vi "EnFlo_Hub.vi"() -> ()   [LabVIEW 2015]
uses:
  Anemometry Sub Vis/Controls/Launch_controls/Open_Calib.ctl
  Anemometry Sub Vis/Controls/Launch_controls/Open_Meas.ctl
  Anemometry Sub Vis/Controls/Launch_controls/Open_Enter_Temp.ctl
  Anemometry Sub Vis/Controls/Launch_controls/Multi_Run_Prog.ctl
  Anemometry Sub Vis/Controls/Launch_controls/EnFlo_arm.ctl
  Anemometry Sub Vis/Controls/Launch_controls/Fast_FID_Valve.ctl
  Anemometry Sub Vis/Controls/Launch_controls/Disp_Setup.ctl
  Anemometry Sub Vis/Controls/Launch_controls/EnFlo_Tun_Setup.ctl
  Anemometry Sub Vis/Controls/Launch_controls/User_Metadata.ctl
  Anemometry Sub Vis/Controls/Launch_controls/Trav_3D_move.ctl
  Anemometry Sub Vis/Controls/Launch_controls/Trav_Space.ctl
  Anemometry Sub Vis/Controls/Launch_controls/Tunnel_speed.ctl
  Anemometry Sub Vis/Controls/Launch_controls/Client_source_control.ctl
  Anemometry Sub Vis/Controls/Launch_controls/Hydrosonic_Manual.ctl
  Anemometry Sub Vis/Controls/Launch_controls/Preference_Panel.ctl
  Anemometry Sub Vis/Controls/Launch_controls/Hot_wire_Calculator.ctl
  Anemometry Sub Vis/Controls/Launch_controls/RW_X_Parker_Config.ctl
  Anemometry Sub Vis/Controls/Launch_controls/LDA_Alignment.ctl
  Anemometry Sub Vis/Controls/Launch_controls/Named_Serial_Comms.ctl
  Anemometry Sub Vis/Controls/Launch_controls/BSA_data_rates.ctl
  Anemometry Sub Vis/Controls/Launch_controls/Serial_Setup.ctl
  Anemometry Sub Vis/Controls/Launch_controls/Post_Process_icon.ctl
  Anemometry Sub Vis/Controls/Launch_controls/Edit_Ascii_file.ctl
  Anemometry Sub Vis/Controls/Launch_controls/Edit_Raw_DF.ctl
  Anemometry Sub Vis/Controls/Launch_controls/Results_file_plotter.ctl
  Anemometry Sub Vis/Controls/Launch_controls/Serial_Port_Names.ctl
  Anemometry Sub Vis/Controls/Launch_controls/Paul.ctl
  Anemometry Sub Vis/Controls/Launch_controls/Tom.ctl
  Anemometry Sub Vis/Controls/Launch_controls/Scani_Valve.ctl
  Anemometry Sub Vis/Controls/Launch_controls/Edit_sever_Channel.ctl
  Anemometry Sub Vis/Controls/Launch_controls/Day_file_plotter.ctl
  Anemometry Sub Vis/Controls/Launch_controls/Plot_Sever_Data.ctl
  Anemometry Sub Vis/Controls/Launch_controls/Adam_Table.ctl
  Anemometry Sub Vis/Controls/Launch_controls/Active_Channel_Control.ctl
  Anemometry Sub Vis/Controls/Launch_controls/Laser on,off.ctl
  Anemometry Sub Vis/Controls/Launch_controls/Laser set power.ctl
  Anemometry Sub Vis/Controls/Preference_Mode.ctl
  Anemometry Sub Vis/Controls/Post_Process.ctl
  Anemometry Sub Vis/Controls/Setup.ctl
  Anemometry Sub Vis/Gen Trav/Trav_mode.ctl
  Anemometry Sub Vis/Controls/User_Specific_mode.ctl
  Anemometry Sub Vis/File/Setup_Filetype.ctl
  Anemometry Sub Vis/Calibration/Calib_mode.ctl
  Anemometry Sub Vis/Controls/Server_Comms.ctl
  ADAM Client/Sub VIs/ADAM Controls/Update_scan_value.ctl
  Anemometry Sub Vis/Controls/App_Global.ctl
  Anemometry Sub Vis/Globals/Meas_global.vi
  Anemometry Sub Vis/Globals/Dynamic_call_global.ph.vi
  Anemometry Sub Vis/Globals/Trav_pos_global.vi
  Anemometry Sub Vis/Globals/Constants_global.vi
  Anemometry Sub Vis/Globals/Preference_global.vi
  Anemometry Sub Vis/Acquisition/PWA/PWAtasksGLOBAL.vi
  <vilib>/Platform/browser.llb/Open URL in Default Browser (string).vi
  Anemometry Sub Vis/Utilities/Email_transfer_global.vi
  Camera Server/Globals/CamServer global.vi
panel:
  out "CamServer machine name or IP":string="EnFlo-CamServer"
  out "List of ADAM channels to view":string[](array[string])
  out "List of ADAM control channels":string[](array[string])
  out "Analogue Dev Name":string="Dev2"
  out "Numeric":i32
  out "Rig Name":string="EnFlo Tunnel"
  out "All Users":path=path "/System Folder/Preferences/LabVIEW (EnFlo specific)/Meas Setups"
  out "Dummy Measurement":bool
  in  "stop":bool
  in  "Tab Control":T1(tab)
  in  "Tunnel Speed Control":T2
  in  "Traverse Space":T3
  in  "Trav 3D Move":T4 caption="3D Traverse Move"
  in  "User Metadata":T5
  in  "Multi Run Prog":T6
  in  "Enter Temp_Press":T7
  in  "Measurement Prog":T8 caption="Measurement"
  in  "Calibration Prog":T9 caption="Calibration"
  in  "Source Live":bool
  in  "Laser set power":T10
  in  "Laser on/off":T11
  in  "Scani Valve":T12
  in  "LDA Alignment":T13
  in  "Hydrosonic Control":T14
  in  "Fast FID Valve":T15
  in  "Source Control":T16
  in  "Gas Release Setup":T17
  in  "EnFlo Tunnel Setup":T18
  in  "Heater Setup":bool caption="Inlet heater File"
  in  "EnFlo Arm":T19
  in  "EnFlo Tun Display":bool
  in  "Beam Check Positions":bool
  in  "Rig_Control":cluster{"Ch Name":string, "Boolean":bool}[](array[cluster])
  in  "ADAM Channels Control":T20 caption="Change Active Channels"
  in  "ADAM Scan Table":T21 caption="Run ADAM Scan Table"
  in  "Edit Server Channel":T22
  in  "Plot Server Channels":T23 caption="Plot Server Data"
  in  "Day Files Plotter":T24 caption="Plot Data From File"
  out "Current Values":cluster{"Ch Name":string, "Numeric":dbl}[](array[cluster])
  in  "Post_Pro_Results_Hierarchy":bool
  in  "Results File Plotter":T25
  in  "Edit Raw Data Files":T26
  in  "Edit ASCII File":T27
  in  "Post Process Raw Data":T28
  in  "Plot_FFID_Calibs.vi":bool
  in  "Top Level Traverse":bool
  in  "Show Manual Sync":bool
  in  "Sync to server now":bool
  in  "Port Names":T29
  in  "Serial Setup":T30
  in  "LDA Data Rate":T31
  in  "Named Serial Comms":T32
  in  "RW Trav Setup":T33
  in  "Hot Wire Calc":T34
  in  "Preference Panel":T35
  in  "Tom Lawton tlawton@cppwind.com":T36 caption="For -other- support"
  in  "Paul Hayden p.hayden@surrey.ac.uk":T37 caption="For software support"
  in  "Online Manual":bool
  out "VI Name":string
  out "Iterations":i32
  # "Or give us a call on Tel: 01483 689545"
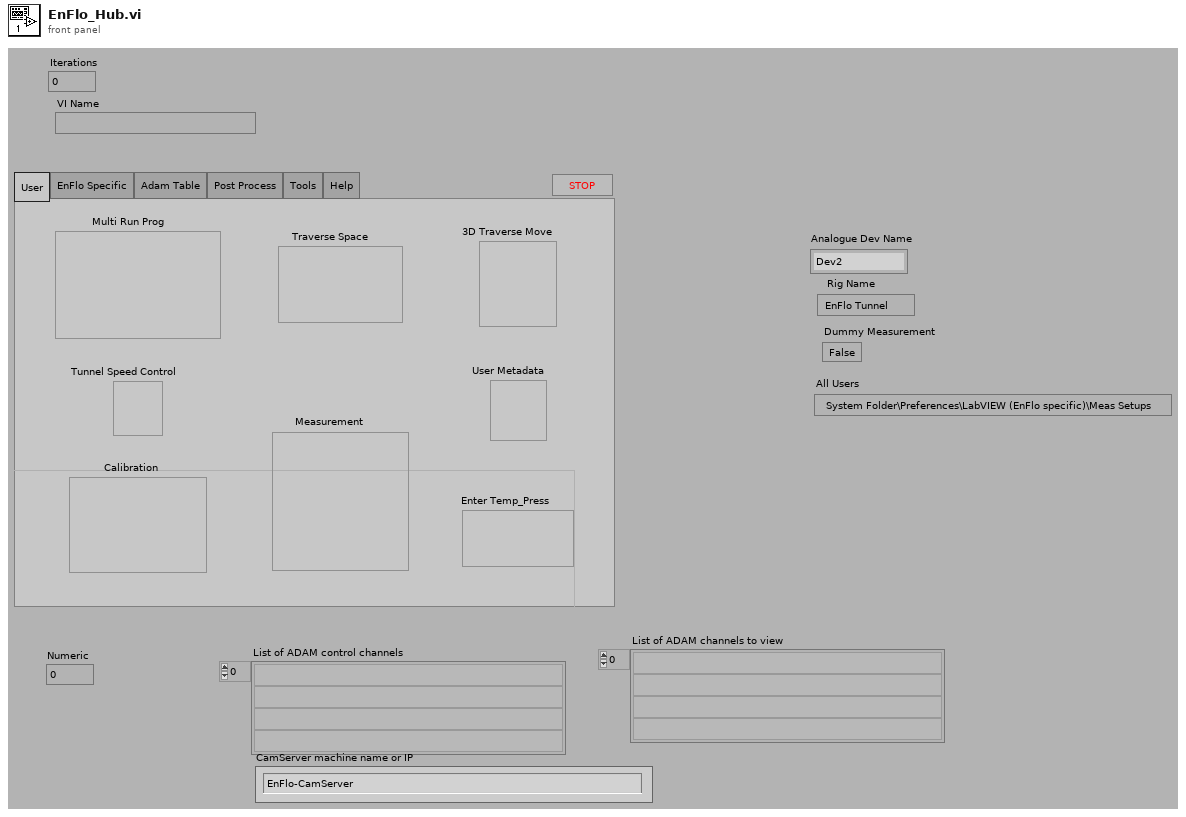
[diagram p1: front panel]
types:
  T1 = enum32{"User", "EnFlo Specific", "Adam Table", "Post Process", "Tools", "Help"}
  T2 = typedef "Tunnel_speed.ctl" = bool
  T3 = typedef "Trav_Space.ctl" = bool
  T4 = typedef "Trav_3D_move.ctl" = bool
  T5 = typedef "User_Metadata.ctl" = bool
  T6 = typedef "Multi_Run_Prog.ctl" = bool
  T7 = typedef "Open_Enter_Temp.ctl" = bool
  T8 = typedef "Open_Meas.ctl" = bool
  T9 = typedef "Open_Calib.ctl" = bool
  T10 = typedef "Laser set power.ctl" = bool
  T11 = typedef "Laser on,off.ctl" = bool
  T12 = typedef "Scani_Valve.ctl" = bool
  T13 = typedef "LDA_Alignment.ctl" = bool
  T14 = typedef "Hydrosonic_Manual.ctl" = bool
  T15 = typedef "Fast_FID_Valve.ctl" = bool
  T16 = typedef "Client_source_control.ctl" = bool
  T17 = typedef "Disp_Setup.ctl" = bool
  T18 = typedef "EnFlo_Tun_Setup.ctl" = bool
  T19 = typedef "EnFlo_arm.ctl" = bool
  T20 = typedef "Active_Channel_Control.ctl" = bool
  T21 = typedef "Adam_Table.ctl" = bool
  T22 = typedef "Edit_sever_Channel.ctl" = bool
  T23 = typedef "Plot_Sever_Data.ctl" = bool
  T24 = typedef "Day_file_plotter.ctl" = bool
  T25 = typedef "Results_file_plotter.ctl" = bool
  T26 = typedef "Edit_Raw_DF.ctl" = bool
  T27 = typedef "Edit_Ascii_file.ctl" = bool
  T28 = typedef "Post_Process_icon.ctl" = bool
  T29 = typedef "Serial_Port_Names.ctl" = bool
  T30 = typedef "Serial_Setup.ctl" = bool
  T31 = typedef "BSA_data_rates.ctl" = bool
  T32 = typedef "Named_Serial_Comms.ctl" = bool
  T33 = typedef "RW_X_Parker_Config.ctl" = bool
  T34 = typedef "Hot_wire_Calculator.ctl" = bool
  T35 = typedef "Preference_Panel.ctl" = bool
  T36 = typedef "Tom.ctl" = bool
  T37 = typedef "Paul.ctl" = bool
  T38 = typedef "Post_Process.ctl" = enum16{"Take New Data", "Post Process Raw Data File"}
  T39 = typedef "Preference_Mode.ctl" = enum16{"Load Preferences from file", "Save Preferences to file", "Load, Edit then Save"}
  T40 = enum32{"User", "EnFlo Lab Specific", "Adam Table", "Post Process", "Tools", "Help"}
  T41 = typedef "Server_Comms.ctl" = enum16{"Server Link Healthy", "Do Not Link To Server"}
  T42 = typedef "Update_scan_value.ctl" = cluster{"Channel Name":string, "New Value":dbl}
  T43 = typedef "Setup.ctl" = enum16{"Run Program", "Show Setup", "Save Current Setup", "Setup Front Panel"}
  T44 = enum16{"Get Channel Names", "Get Current Value", "Update Channel Value", "Update Channel Description"}
  T45 = enum32{"Invalid", "Standard", "Closed", "Hidden", "Minimized", "Maximized"}
  T46 = enum32{"Bad", "Idle", "Run top level", "Running"}
  T47 = enum16{"Load From Excel File", "Save to Excel File"}
  T48 = typedef "User_Specific_mode.ctl" = enum16{"Check VI only", "Run VI"}
  T49 = typedef "Trav_mode.ctl" = enum16{"Move traverse", "Read traverse position", "Teach Position"}
  T50 = typedef "Setup_Filetype.ctl" = enum16{"Measurement Setups", "Calibration Setups", "General", "Results File Plotter Setups", "Speed Calib Tweaks"}
  T51 = enum16{"Load Command File", "Save Command File", "Check Multi Run Prog", "Check Multi Run Prog With Live Moves", "Run Multi Run Prog"}
  T52 = typedef "Calib_mode.ctl" = enum16{"Show Setup", "Take a New Calibration Point", "Refit Curve", "Setup Front Panel"}
  T53 = typedef "App_Global.ctl" = enum16{"Read Global", "Write to Global", "Initialise Array"}
  T54 = typedef "Tunnel_Coordinates.ctl" = enum16{"Work in Tunnel Coordinates", "Work in Model Coordinates"}
  T55 = typedef "App_Ref_Cluster.ctl" = cluster{"Server IP & Port No":string, "Application reference":refnum<vi>}
  T56 = typedef "Ch_description_ADAM.ctl" = cluster{"Ch Name":string, "Type":T57, "Function":T58, "Ch State":T59, "Calibration type":T60, "A":dbl, "B":dbl, "C":dbl, "D":dbl, "Comments":string, "Address":T61, "String":string, "Duty":u16}
  T57 = typedef "Module_type_ADAM.ctl" = string
  T58 = typedef "Function_ADAM.ctl" = enum16{"Analogue Input", "Digital Input", "Event counter", "Event rate", "Analogue Output", "Digital Output", "Relay Output"}
  T59 = typedef "Channel_State.ctl" = enum16{"On", "Off", "Always On", "Always Off"}
  T60 = typedef "Calib_type_ADAM.ctl" = enum16{"Raw", "Bx + A", "Cx^2 + Bx + A", "Dx^3 + Cx^2 + Bx + A", "In Band", "Hi-Tec Q", "Hi-Tec M_dot", "Text"}
  T61 = typedef "Address.ctl" = cluster{"Main":i32, "Ch.":i32, "Sub":i32, "Port Name":string}
  T62 = typedef "Monitor values.ctl" = cluster{"Power (mW)":sgl, "LDD current (A)":sgl, "TEC drive (V)":sgl, "TEC temp. (degC)":sgl, "SHG heater (degC)":sgl, "BRF heater (degC)":sgl}
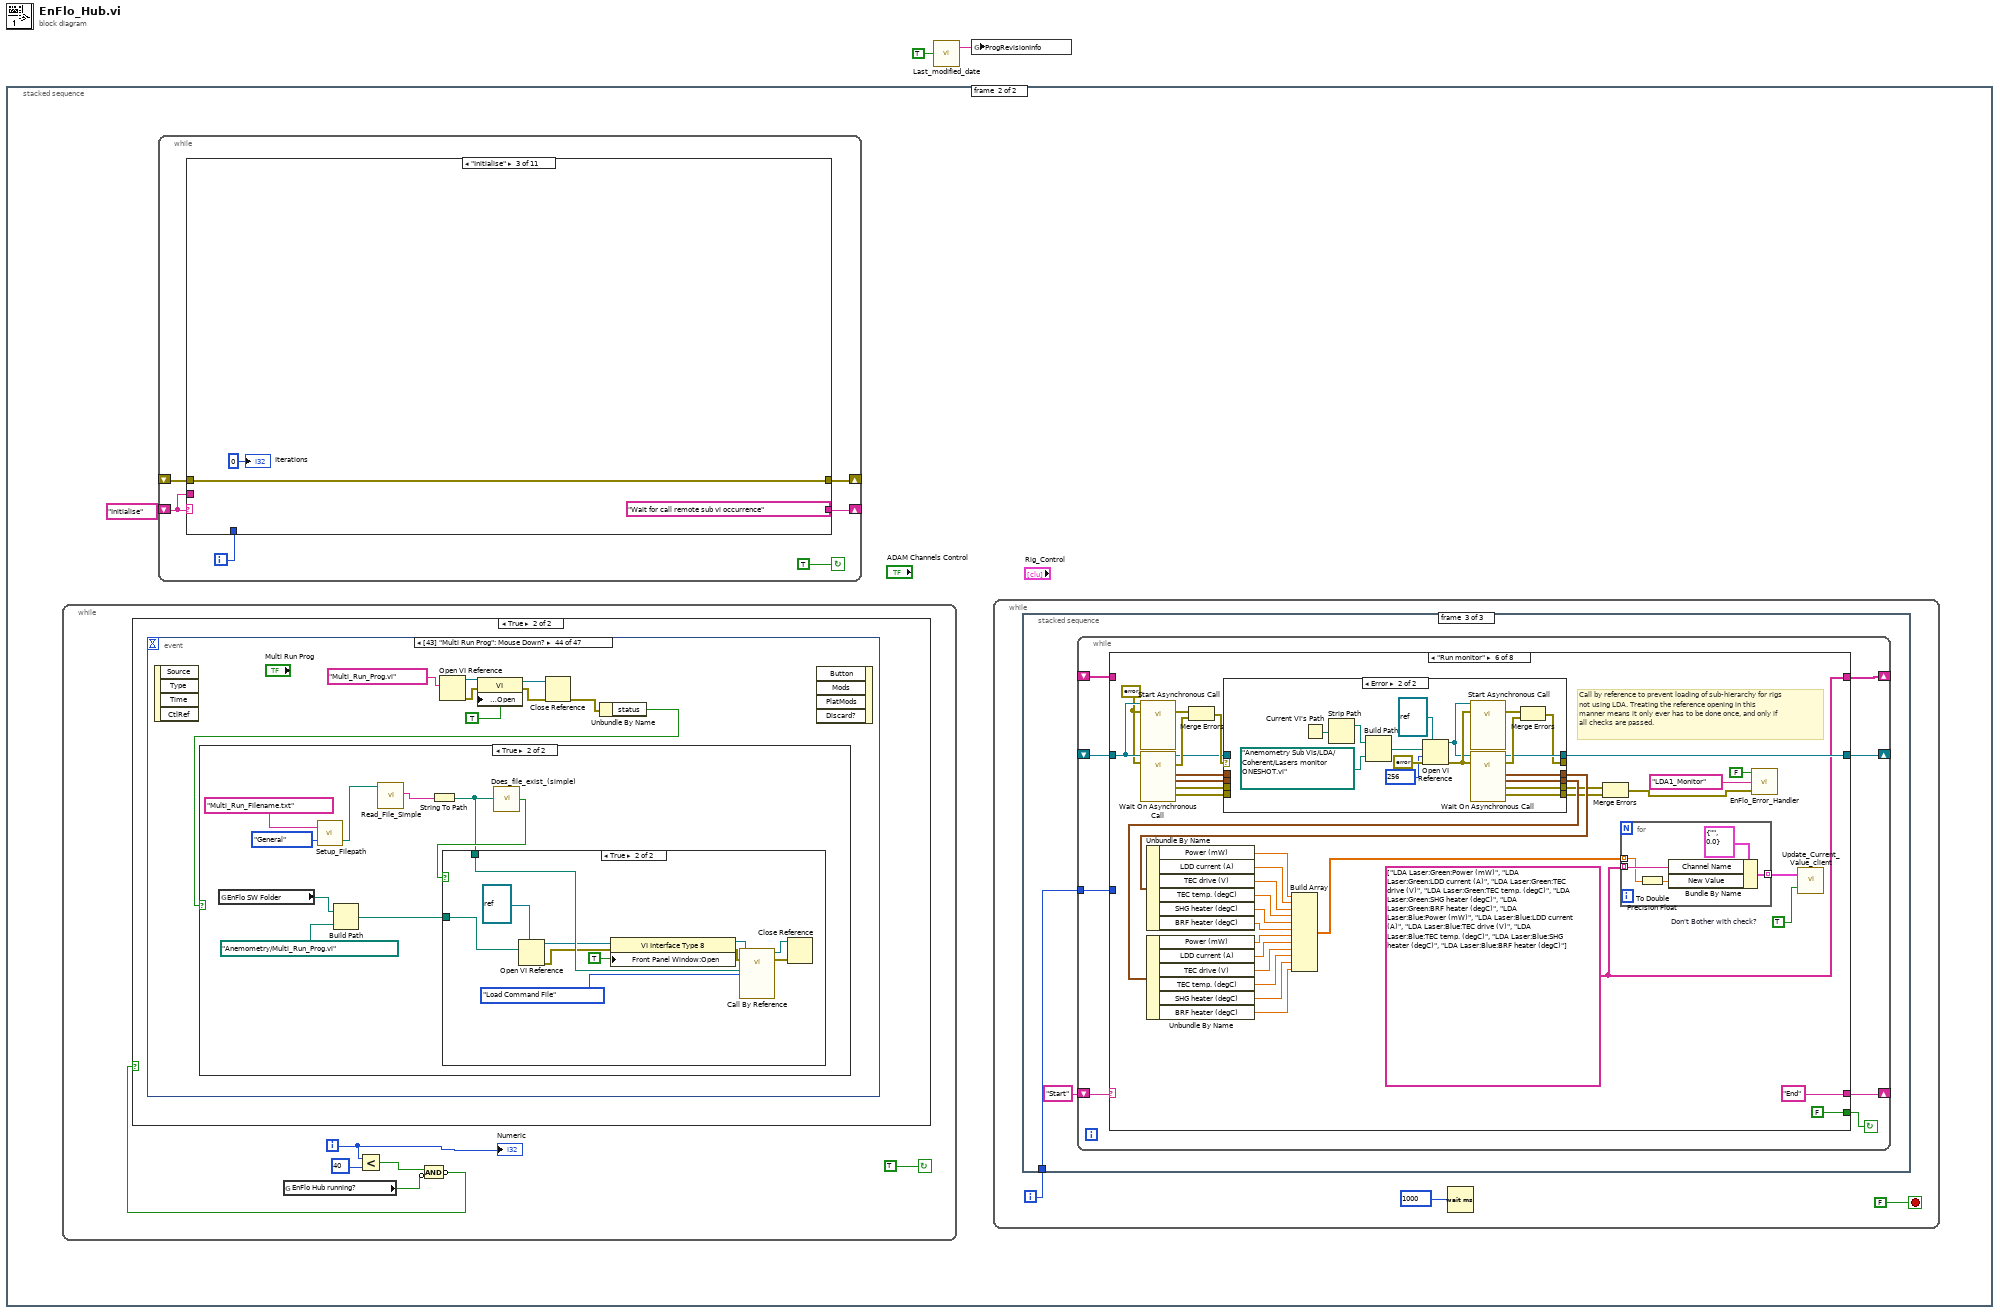
[diagram p0: block diagram]
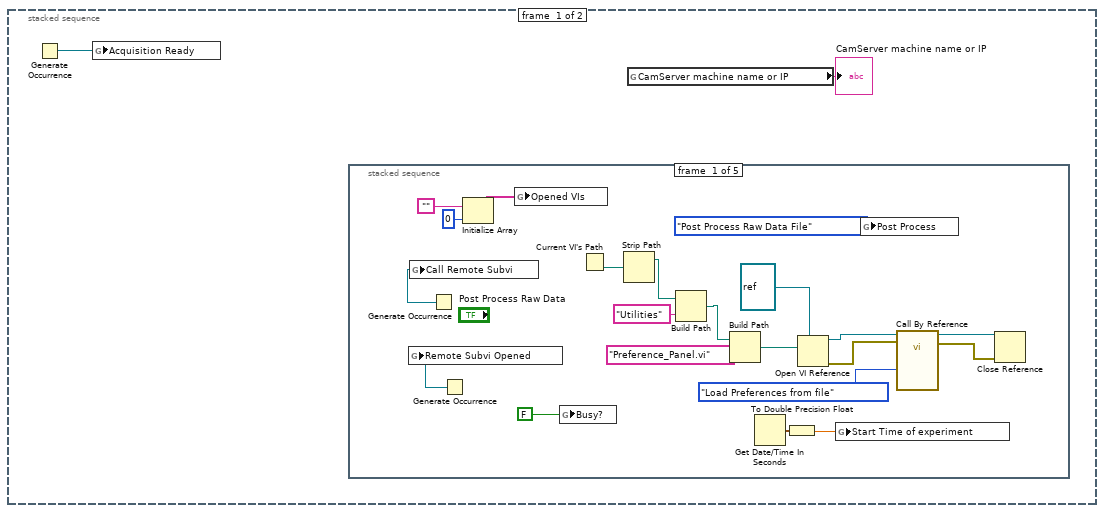
[diagram p2: hidden frame]
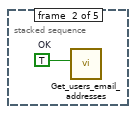
[diagram p3: hidden frame]
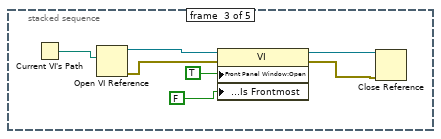
[diagram p4: hidden frame]
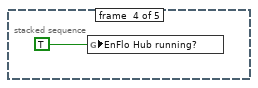
[diagram p5: hidden frame]
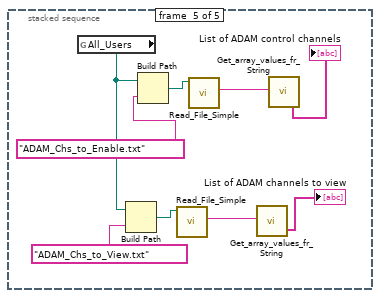
[diagram p6: hidden frame]
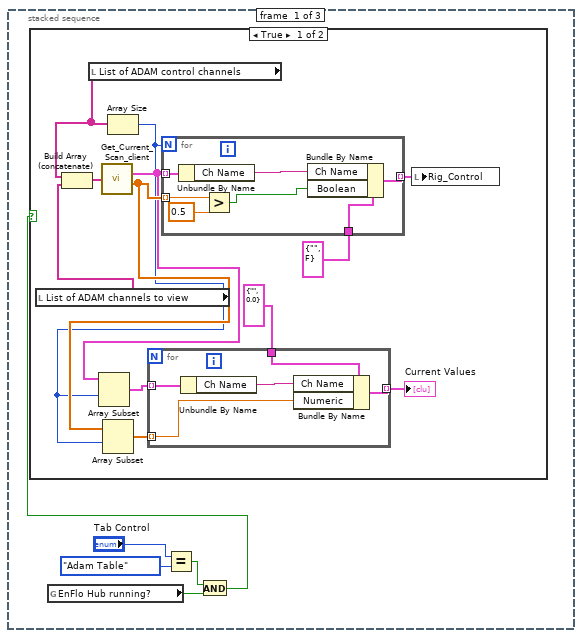
[diagram p7: hidden frame]
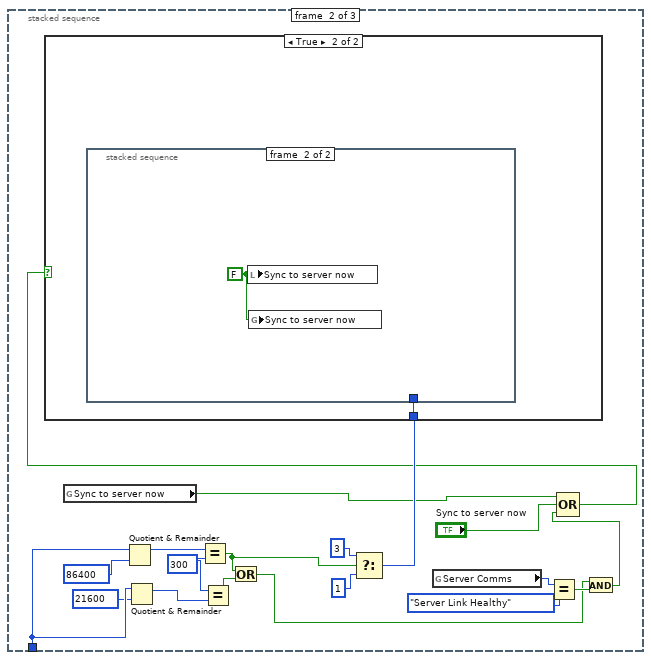
[diagram p9: hidden frame]
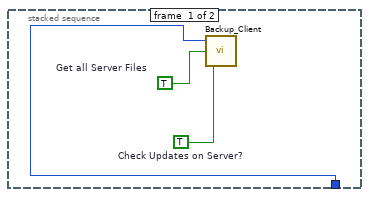
[diagram p11: hidden frame]
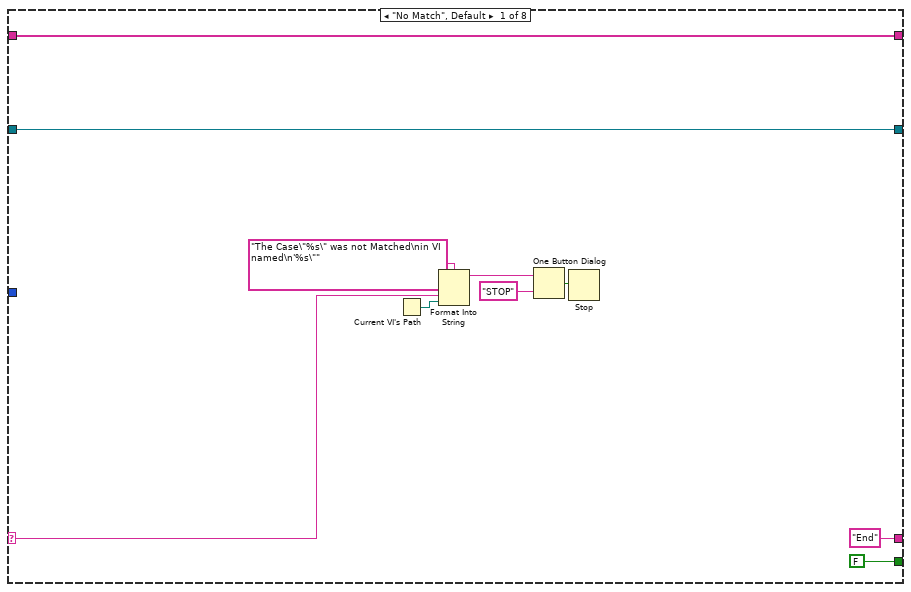
[diagram p12: hidden frame]
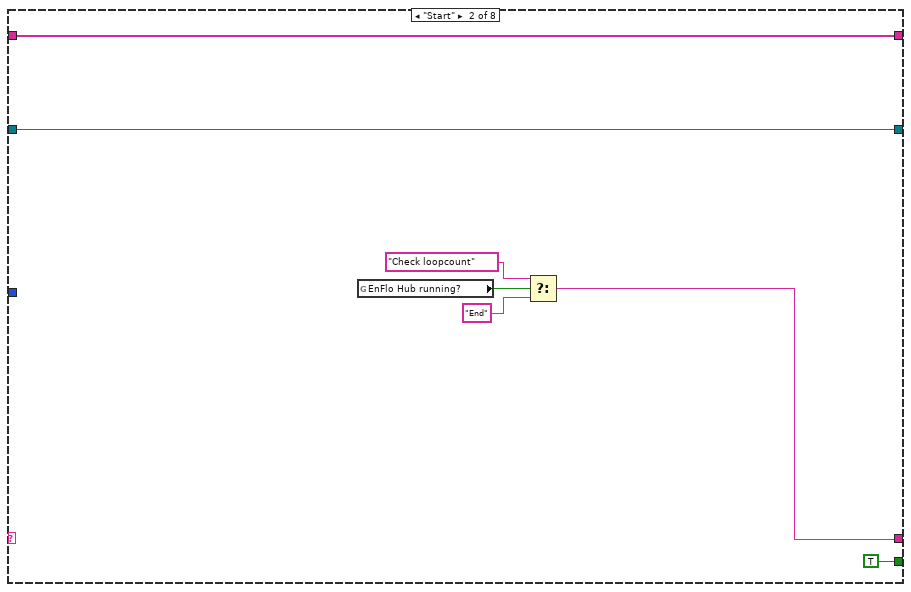
[diagram p13: hidden frame]
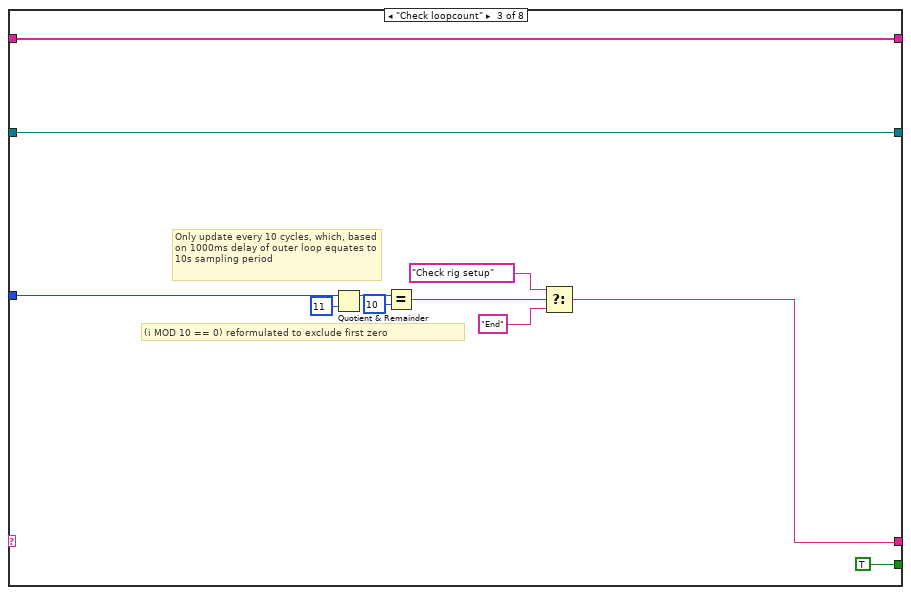
[diagram p14: hidden frame]
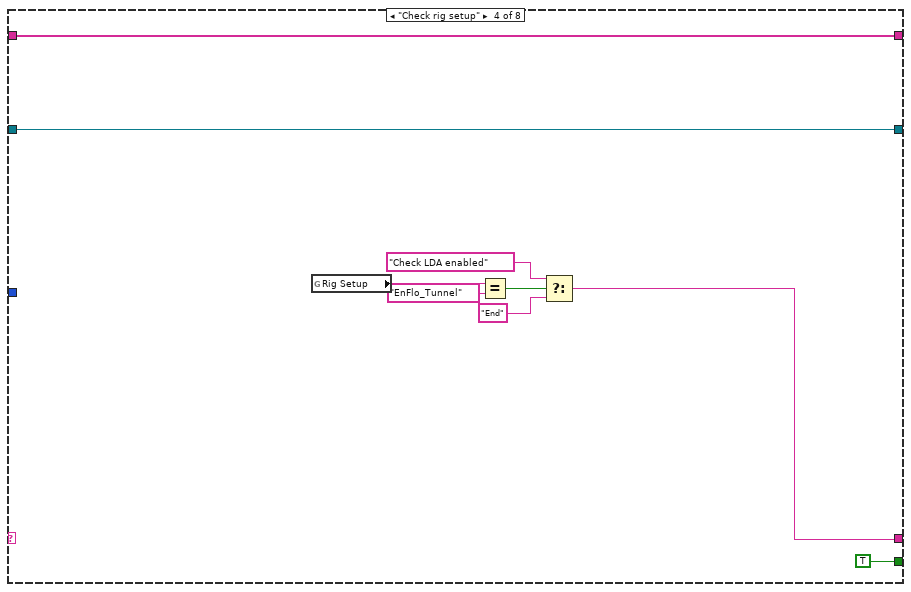
[diagram p15: hidden frame]
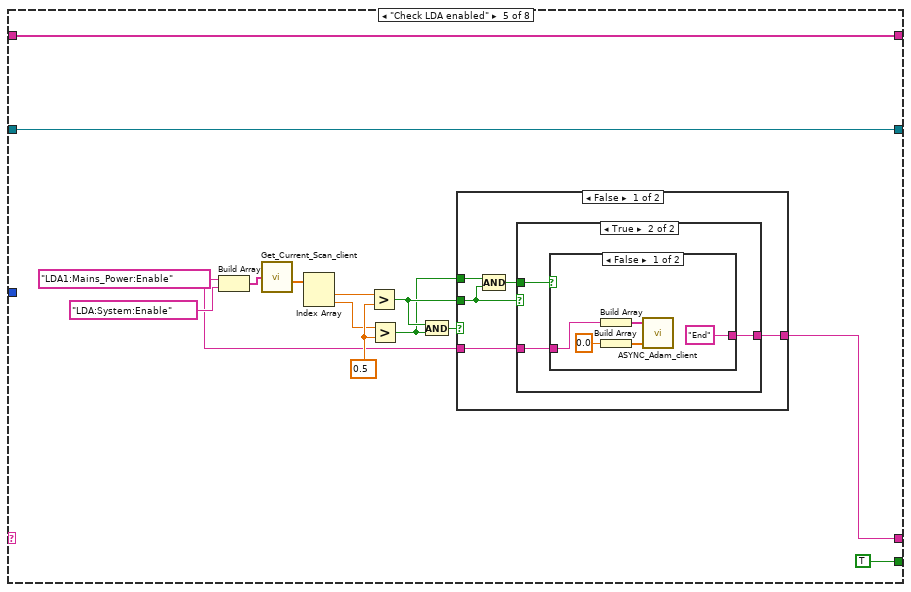
[diagram p16: hidden frame]
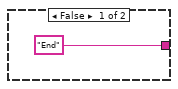
[diagram p17: hidden frame]
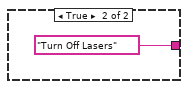
[diagram p18: hidden frame]
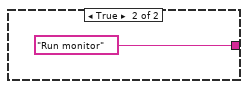
[diagram p19: hidden frame]
diagram:
  n1 = stacked-sequence {
    frame #0 {
      n2 = Generate Occurrence() -> (w4:refnum<k4>)
      n3 = global write "Meas_global.vi" "Acquisition Ready"(w4) -> ()
      n4 = stacked-sequence {
        frame #0 {
          n5 = Generate Occurrence() -> (w25:refnum<k4>)
          n6 = global write "Dynamic_call_global.ph.vi" "Call Remote Subvi"(w25) -> ()
          n7 = Generate Occurrence() -> (w24:refnum<k4>)
          n8 = global write "Dynamic_call_global.ph.vi" "Remote Subvi Opened"(w24) -> ()
          n9 = Initialize Array("", 0) -> (w22:string[])
          n10 = global write "Dynamic_call_global.ph.vi" "Opened VIs"(w22) -> ()
          n11 = global write "Email_transfer_global.vi" "Busy?"(FALSE ("Busy?")) -> ()
          n12 = Current VI's Path() -> (path=w14:path)
          n13 = Strip Path(path=w14) -> (stripped path=w12:path)  [unwired: 1 out]
          n14 = Build Path(base path=w12, name or relative path="Utilities") -> (appended path=w10:path)
          n15 = Build Path(base path=w10, name or relative path="Preference_Panel.vi") -> (appended path=w9:path)
          n16 = Get Date/Time In Seconds() -> (seconds since 1Jan1904=w20:timestamp)
          n17 = To Double Precision Float(number=w20) -> (double precision float=w19:dbl)
          n18 = Open VI Reference(type specifier VI Refnum (for type only)=refnum<vi> refnum, vi path=w9) -> (vi reference=w15:refnum<vi>, error out=w16:errorcluster)  [unwired: 1 in, 3 out]
          n19 = global write "Meas_global.vi" "Start Time of experiment"(w19) -> ()
          n20 = global write "Meas_global.vi" "Post Process"(Post_Process."Post Process Raw Data File" ("Post Process")) -> ()
          n21 = call-by-ref "?"(reference=w15, error in=w16, "Mode"=Preference_Mode."Load Preferences from file") -> (reference out=w17:refnum<vi>, error out=w18:errorcluster)
          n22 = Close Reference(reference=w17, error in (no error)=w18) -> ()  [unwired: 1 out]
        }
        frame #1 {
          w26 = TRUE  # OK
          n23 = call "Get_users_email_addresses.vi"("OK"=w26) -> ()  [unwired: 5 out]
        }
        frame #2 {
          n24 = Current VI's Path() -> (path=w33:path)
          n25 = Open VI Reference(vi path=w33) -> (vi reference=w32:refnum<vi>, error out=w31:errorcluster)  [unwired: 1 in, 4 out]
          n26 = property class="VI"(reference=w32, error in=w31, "Front Panel Window:Open"=TRUE, "Front Panel Window:Is Frontmost"=FALSE) -> (reference out=w30:refnum<vi>, error out=w29:errorcluster)
          n27 = Close Reference(reference=w30, error in (no error)=w29) -> ()  [unwired: 1 out]
        }
        frame #3 {
          n28 = global write "Dynamic_call_global.ph.vi" "EnFlo Hub running?"(TRUE ("EnFlo Hub running?")) -> ()
        }
        frame #4 {
          n29 = global read "Constants_global.vi" "All_Users"() -> (w38:path)
          n30 = Build Path(base path=w38, name or relative path="ADAM_Chs_to_View.txt") -> (appended path=w40:path)
          n31 = Build Path(base path=w38, name or relative path="ADAM_Chs_to_Enable.txt") -> (appended path=w42:path)
          n32 = call "Read_File_Simple.vi"("Filename"=w40) -> ("string"=w39:string)  [unwired: 2 in, 7 out]
          n33 = call "Read_File_Simple.vi"("Filename"=w42) -> ("string"=w43:string)  [unwired: 2 in, 7 out]
          n34 = call "Get_array_values_fr_String.vi"("String Value"=w39) -> ("String array"=→"List of ADAM channels to view":string[])  [unwired: 1 out]
          n35 = call "Get_array_values_fr_String.vi"("String Value"=w43) -> ("String array"=→"List of ADAM control channels":string[])  [unwired: 1 out]
        }
      }
      n36 = global read "CamServer global.vi" "CamServer machine name or IP"() -> (→"CamServer machine name or IP":string)
    }
    frame #1 {
      n37 = while {
        i -> [w272]
        stop <- TRUE continue-if-true
        n38 = global read "Dynamic_call_global.ph.vi" "EnFlo Hub running?"() -> (w270:bool)
        n39 = Less?(x=w272, y=40) -> (x < y?=w269:bool)
        n40 = Compound Arithmetic op=AND(w269, invert w270) -> (invert w268:bool)
        n41 = case shown="True" w268 {
          frame False {
            n42 = Wait (ms)(milliseconds to wait=u32 200) -> ()  [unwired: 1 out]
          }
          frame True {
            n43 = event shown="[43] \"Multi Run Prog\": Mouse Down?" {
              selector: _ -> [_ _ _ _ _ _ _ _ _ _ _ _ _ _ _ _ _ _ _ _ _ _ _ _ _ _ _ _ _ _ _ _ _ _ _ _ _ _ _ _ _ _ _ _ _ _ _]
              dyn-events: _ -> [_ _ _ _ _ _ _ _ _ _ _ _ _ _ _ _ _ _ _ _ _ _ _ _ _ _ _ _ _ _ _ _ _ _ _ _ _ _ _ _ _ _ _ _ _ _ _]
              timeout: _ -> [_ _ _ _ _ _ _ _ _ _ _ _ _ _ _ _ _ _ _ _ _ _ _ _ _ _ _ _ _ _ _ _ _ _ _ _ _ _ _ _ _ _ _ _ _ _ _]
              event Mouse Down? {
                w283 = "Measurement.vi" ("name or relative path")
                n44 = event-data() -> ()  [unwired: 2 out]
                n45 = global read "Constants_global.vi" "EnFlo SW Folder"() -> (w286:path)
                n46 = Open VI Reference(vi path=w283) -> (vi reference=w282:refnum<vi>, error out=w281:errorcluster)  [unwired: 1 in, 4 out]
                n47 = Build Path(base path=w286, name or relative path="Anemometry") -> (appended path=w289:path)
                n48 = property class="VI"(reference=w282, error in=w281, "Front Panel Window:Open"=TRUE) -> (reference out=w279:refnum<vi>, error out=w280:errorcluster)
                n49 = Build Path(base path=w289, name or relative path=w283) -> (appended path=w287:path)
                n50 = global read "Preference_global.vi" "Rig Setup"() -> (w277:string)
                n51 = Close Reference(reference=w279, error in (no error)=w280) -> (error out=w278:errorcluster)
                n52 = Unbundle By Name(w278) -> ("status"=w288:bool)
                n53 = Equal?(x="Post_Processing_Machine" ("Rig Setup"), y=w277) -> (x = y?=w275:bool)
                n54 = case shown="True" w288 {
                  tunnel: w287 -> [_ w292]
                  tunnel: w278 -> [_ _]
                  tunnel: w275 -> [_ w291]
                  frame False {
                  }
                  frame True {
                    n55 = stacked-sequence {
                      tunnel: w292 -> [w302 _]
                      tunnel: w291 -> [w293 _]
                      frame #0 {
                        n56 = Open VI Reference(type specifier VI Refnum (for type only)=refnum<vi> refnum, vi path=w302) -> (vi reference=w300:refnum<vi>, error out=w299:errorcluster)  [unwired: 1 in, 3 out]
                        n57 = property class="VI Interface Type 1"(reference=w300, error in=w299, "Front Panel Window:Open"=TRUE) -> (reference out=w295:refnum<vi>, error out=w294:errorcluster)
                        n58 = case shown="False" w293 {
                          tunnel: [w308 w310] -> w298
                          tunnel: [w307 w309] -> w297
                          tunnel: w295 -> [w306 w310]
                          tunnel: w294 -> [w305 w309]
                          frame False {
                            n59 = call-by-ref "?"(reference=w306, error in=w305, "setup"=Setup."Setup Front Panel", "Post Process"=Post_Process."Take New Data") -> (reference out=w308:refnum<vi>, error out=w307:errorcluster)  [unwired: 16 in, 2 out]
                          }
                          frame True {
                          }
                        }
                        n60 = Close Reference(reference=w298, error in (no error)=w297) -> ()  [unwired: 1 out]
                      }
                      frame #1 {
                        n61 = global write "Meas_global.vi" "Post Process"(Post_Process."Post Process Raw Data File" ("Post Process")) -> ()
                      }
                    }
                  }
                }
                n62 = event-data("Discard?"=TRUE) -> ()  [unwired: 1 in, 2 out]
              }
              event Mouse Down? {
                n63 = event-data() -> ()  [unwired: 2 out]
                n64 = call-poly <vilib>:"Open URL in Default Browser.vi"("URL"="Mailto:tlawton@cppwind.com") -> ()  [unwired: 1 in, 6 out]
                n65 = event-data() -> ()  [unwired: 1 in, 5 out]
              }
              event Mouse Down? {
                n66 = event-data() -> ()  [unwired: 5 out]
                n67 = call-poly <vilib>:"Open URL in Default Browser.vi"("URL"="Mailto:p.hayden@surrey.ac.uk") -> ()  [unwired: 1 in, 6 out]
                n68 = event-data() -> ()  [unwired: 1 in, 2 out]
              }
              event "Online Manual": Mouse Down? {
                n69 = event-data() -> ()  [unwired: 2 out]
                n70 = call-poly <vilib>:"Open URL in Default Browser.vi"("URL"="http://131.227.181.18/~xphayden/enflosw/beta/Manual/online/index.html") -> ()  [unwired: 1 in, 6 out]
                n71 = event-data() -> ()  [unwired: 1 in, 2 out]
              }
              event Mouse Down? {
                n72 = event-data() -> ()  [unwired: 9 out]
                n73 = global read "Constants_global.vi" "EnFlo SW Folder"() -> (w315:path)
                n74 = Build Path(base path=w315, name or relative path=path "ADAM Client/ADAM client VIs/ScaniValve_client.vi") -> (appended path=w318:path)
                n75 = call "Open_Close_Front_Panel.ph.vi"("Front Panel Window:Open"=TRUE, "VI path"=w318) -> ()  [unwired: 2 out]
                n76 = event-data() -> ()  [unwired: 1 in, 5 out]
              }
              event Mouse Down? {
                n77 = event-data() -> ()  [unwired: 9 out]
                n78 = global read "Constants_global.vi" "EnFlo SW Folder"() -> (w319:path)
                n79 = Build Path(base path=w319, name or relative path=path "Anemometry/Anemometry Sub Vis/LDA/Coherent/Laser power on,off (simple).vi") -> (appended path=w322:path)
                n80 = call "Open_Close_Front_Panel.ph.vi"("Front Panel Window:Open"=TRUE, "VI path"=w322) -> ()  [unwired: 2 out]
                n81 = event-data() -> ()  [unwired: 2 in, 1 out]
              }
              event "Source Live": Value Change {
                n82 = event-data() -> ()  [unwired: 7 out]
                n83 = flat-sequence {
                  frame #0 {
                    n84 = global read "Constants_global.vi" "EnFlo SW Folder"() -> (w323:path)
                    n85 = Build Path(base path=w323, name or relative path=path "ADAM Serial/Instrument drivers/Arduino/Source_Live_Control.vi") -> (appended path=w326:path)
                    n86 = call "Open_Close_Front_Panel.ph.vi"("Front Panel Window:Open"=TRUE, "VI path"=w326) -> ()  [unwired: 2 out]
                  }
                  frame #1 {
                    n87 = local write "Source Live"(FALSE) -> ()
                  }
                }
              }
              event Mouse Down? {
                n88 = event-data() -> ()  [unwired: 9 out]
                n89 = global read "Constants_global.vi" "EnFlo SW Folder"() -> (w328:path)
                n90 = Build Path(base path=w328, name or relative path=path "Anemometry/Anemometry Sub Vis/LDA/Coherent/Set lasers power.vi") -> (appended path=w331:path)
                n91 = call "Open_Close_Front_Panel.ph.vi"("Front Panel Window:Open"=TRUE, "VI path"=w331) -> ()  [unwired: 2 out]
                n92 = event-data() -> ()  [unwired: 2 in, 1 out]
              }
              event Mouse Down? {
                n93 = event-data() -> ()  [unwired: 5 out]
                n94 = global read "Constants_global.vi" "EnFlo SW Folder"() -> (w332:path)
                n95 = Build Path(base path=w332, name or relative path=path "ADAM Client/ADAM client VIs/Day_File_Plotter.vi") -> (appended path=w338:path)
                n96 = Open VI Reference(vi path=w338) -> (vi reference=w339:refnum<vi>, error out=w341:errorcluster)  [unwired: 2 in, 3 out]
                n97 = property class="VI"(reference=w339, error in=w341, "Front Panel Window:Open"=TRUE) -> (reference out=w343:refnum<vi>, error out=w342:errorcluster)
                n98 = invoke class="VI" method="Run VI"(reference=w343, error in=w342, "Wait until done"=FALSE, "Auto Dispose Ref"=TRUE) -> (reference out=w334:refnum<vi>, error out=w335:errorcluster)  [unwired: 1 in, 3 out]
                n99 = Close Reference(reference=w334, error in (no error)=w335) -> ()  [unwired: 1 out]
                n100 = event-data() -> ()  [unwired: 1 in, 4 out]
              }
              event Mouse Down? {
                n101 = event-data() -> ()  [unwired: 5 out]
                n102 = global read "Constants_global.vi" "EnFlo SW Folder"() -> (w344:path)
                n103 = Build Path(base path=w344, name or relative path=path "ADAM Serial/Serial Link Layer/Port_Names.vi") -> (appended path=w346:path)
                n104 = Open VI Reference(vi path=w346) -> (vi reference=w351:refnum<vi>, error out=w352:errorcluster)  [unwired: 1 in, 4 out]
                n105 = invoke class="VI" method="Run VI"(reference=w351, error in=w352, "Wait until done"=TRUE, "Auto Dispose Ref"=TRUE) -> (reference out=w347:refnum<vi>, error out=w348:errorcluster)  [unwired: 1 in, 3 out]
                n106 = Close Reference(reference=w347, error in (no error)=w348) -> ()  [unwired: 1 out]
                n107 = event-data() -> ()  [unwired: 1 in, 5 out]
              }
              event Mouse Down? {
                n108 = event-data() -> ()  [unwired: 5 out]
                n109 = global read "Constants_global.vi" "EnFlo SW Folder"() -> (w353:path)
                n110 = Build Path(base path=w353, name or relative path=path "Data plotting/Results_file_Plotter.vi") -> (appended path=w356:path)
                n111 = Open VI Reference(vi path=w356) -> (vi reference=w358:refnum<vi>, error out=w355:errorcluster)  [unwired: 1 in, 4 out]
                n112 = property class="VI"(reference=w358, error in=w355, "Front Panel Window:Open"=TRUE) -> (reference out=w359:refnum<vi>, error out=w360:errorcluster)
                n113 = invoke class="VI" method="Run VI"(reference=w359, error in=w360, "Wait until done"=FALSE, "Auto Dispose Ref"=TRUE) -> (reference out=w361:refnum<vi>, error out=w362:errorcluster)  [unwired: 1 in, 3 out]
                n114 = Close Reference(reference=w361, error in (no error)=w362) -> ()  [unwired: 1 out]
                n115 = event-data() -> ()  [unwired: 1 in, 5 out]
              }
              event Mouse Down? {
                n116 = event-data() -> ()  [unwired: 5 out]
                n117 = global read "Constants_global.vi" "EnFlo SW Folder"() -> (w365:path)
                n118 = Build Path(base path=w365, name or relative path=path "Anemometry/Utilities/Post_Process_Raw_data.vi") -> (appended path=w367:path)
                n119 = call "Open_Close_Front_Panel.ph.vi"("Front Panel Window:Open"=TRUE, "VI path"=w367) -> ()  [unwired: 2 out]
                n120 = event-data() -> ()  [unwired: 1 in, 5 out]
              }
              event Mouse Down? {
                n121 = event-data() -> ()  [unwired: 5 out]
                n122 = global read "Constants_global.vi" "EnFlo SW Folder"() -> (w369:path)
                n123 = Build Path(base path=w369, name or relative path=path "Anemometry/Anemometry Sub Vis/Data_plotting_vis/Edit_Raw_DF_Header.vi") -> (appended path=w371:path)
                n124 = call "Open_Close_Front_Panel.ph.vi"("Front Panel Window:Open"=TRUE, "VI path"=w371) -> ()  [unwired: 2 out]
                n125 = event-data() -> ()  [unwired: 1 in, 5 out]
              }
              event Mouse Down? {
                n126 = event-data() -> ()  [unwired: 5 out]
                n127 = global read "Constants_global.vi" "EnFlo SW Folder"() -> (w373:path)
                n128 = Build Path(base path=w373, name or relative path=path "ADAM Serial/Serial Link Layer/Serial_Setup.vi") -> (appended path=w375:path)
                n129 = Open VI Reference(vi path=w375) -> (vi reference=w380:refnum<vi>, error out=w381:errorcluster)  [unwired: 1 in, 4 out]
                n130 = invoke class="VI" method="Run VI"(reference=w380, error in=w381, "Wait until done"=TRUE, "Auto Dispose Ref"=TRUE) -> (reference out=w376:refnum<vi>, error out=w377:errorcluster)  [unwired: 1 in, 3 out]
                n131 = Close Reference(reference=w376, error in (no error)=w377) -> ()  [unwired: 1 out]
                n132 = event-data() -> ()  [unwired: 1 in, 2 out]
              }
              event Mouse Down? {
                n133 = event-data() -> ()  [unwired: 5 out]
                n134 = global read "Constants_global.vi" "EnFlo SW Folder"() -> (w383:path)
                n135 = Build Path(base path=w383, name or relative path=path "ADAM Serial/Serial Link Layer/Named_Serial_Comms.vi") -> (appended path=w385:path)
                n136 = call "Open_Close_Front_Panel.ph.vi"("Front Panel Window:Open"=TRUE, "VI path"=w385) -> ()  [unwired: 2 out]
                n137 = event-data() -> ()  [unwired: 1 in, 5 out]
              }
              event Mouse Down? {
                n138 = event-data() -> ()  [unwired: 5 out]
                n139 = global read "Constants_global.vi" "EnFlo SW Folder"() -> (w386:path)
                n140 = Build Path(base path=w386, name or relative path=path "Anemometry/Anemometry Sub Vis/LDA/LDA_data_rate.vi") -> (appended path=w388:path)
                n141 = call "Open_Close_Front_Panel.ph.vi"("Front Panel Window:Open"=TRUE, "VI path"=w388) -> ()  [unwired: 2 out]
                n142 = event-data() -> ()  [unwired: 1 in, 2 out]
              }
              event Mouse Down? {
                n143 = event-data() -> ()  [unwired: 5 out]
                n144 = global read "Constants_global.vi" "EnFlo SW Folder"() -> (w400:path)
                n145 = Build Path(base path=w400, name or relative path=path "ADAM Client/ADAM client VIs/Control_Channel_Status.vi") -> (appended path=w390:path)
                n146 = Open VI Reference(vi path=w390) -> (vi reference=w393:refnum<vi>, error out=w391:errorcluster)  [unwired: 1 in, 4 out]
                n147 = property class="VI"(reference=w393, error in=w391, "Front Panel Window:Open"=TRUE) -> (reference out=w394:refnum<vi>, error out=w395:errorcluster)
                n148 = invoke class="VI" method="Run VI"(reference=w394, error in=w395, "Wait until done"=FALSE, "Auto Dispose Ref"=TRUE) -> (reference out=w396:refnum<vi>, error out=w397:errorcluster)  [unwired: 1 in, 3 out]
                n149 = Close Reference(reference=w396, error in (no error)=w397) -> ()  [unwired: 1 out]
                n150 = event-data() -> ()  [unwired: 1 in, 2 out]
              }
              event Mouse Down? {
                n151 = event-data() -> ()  [unwired: 5 out]
                n152 = global read "Constants_global.vi" "EnFlo SW Folder"() -> (w402:path)
                n153 = Build Path(base path=w402, name or relative path=path "Anemometry/Utilities/LDA_Beam_Alignment.vi") -> (appended path=w404:path)
                n154 = call "Open_Close_Front_Panel.ph.vi"("Front Panel Window:Open"=TRUE, "VI path"=w404) -> ()  [unwired: 2 out]
                n155 = event-data() -> ()  [unwired: 1 in, 5 out]
              }
              event Mouse Down? {
                w407 = FALSE  # Wait until done
                n156 = event-data() -> ()  [unwired: 5 out]
                n157 = call "Run_Enter_Temp.vi"("Wait until done"=w407) -> ()  [unwired: 1 out]
                n158 = event-data("Discard?"=TRUE) -> ()  [unwired: 1 in, 4 out]
              }
              event Mouse Down? {
                n159 = event-data() -> ()  [unwired: 5 out]
                n160 = global read "Constants_global.vi" "EnFlo SW Folder"() -> (w408:path)
                n161 = Build Path(base path=w408, name or relative path=path "Anemometry/Utilities/Edit_ASCI_file.vi") -> (appended path=w411:path)
                n162 = call "Open_Close_Front_Panel.ph.vi"("Front Panel Window:Open"=TRUE, "VI path"=w411) -> ()  [unwired: 2 out]
                n163 = event-data() -> ()  [unwired: 1 in, 5 out]
              }
              event "Heater Setup": Mouse Down? {
                n164 = event-data() -> ()  [unwired: 5 out]
                n165 = global read "Constants_global.vi" "EnFlo SW Folder"() -> (w412:path)
                n166 = Build Path(base path=w412, name or relative path=path "Anemometry/Utilities/Create_Heater_Setpoints_File.vi") -> (appended path=w415:path)
                n167 = call "Open_Close_Front_Panel.ph.vi"("Front Panel Window:Open"=TRUE, "VI path"=w415) -> ()  [unwired: 2 out]
                n168 = event-data() -> ()  [unwired: 1 in, 5 out]
              }
              event Mouse Down? {
                n169 = event-data() -> ()  [unwired: 5 out]
                n170 = global read "Constants_global.vi" "EnFlo SW Folder"() -> (w416:path)
                n171 = Build Path(base path=w416, name or relative path=path "ADAM Client/Sub VIs/Gas_Release_Control.vi") -> (appended path=w419:path)
                n172 = call "Open_Close_Front_Panel.ph.vi"("Front Panel Window:Open"=TRUE, "VI path"=w419) -> ()  [unwired: 2 out]
                n173 = event-data() -> ()  [unwired: 1 in, 5 out]
              }
              event Mouse Down? {
                n174 = event-data() -> ()  [unwired: 5 out]
                n175 = global read "Constants_global.vi" "EnFlo SW Folder"() -> (w420:path)
                n176 = Build Path(base path=w420, name or relative path=path "ADAM Client/ADAM client VIs/Edit_Server_Channel.vi") -> (appended path=w430:path)
                n177 = Open VI Reference(type specifier VI Refnum (for type only)=refnum<vi> refnum, vi path=w430) -> (vi reference=w423:refnum<vi>, error out=w424:errorcluster)  [unwired: 1 in, 3 out]
                n178 = property class="VI Interface Type 2"(reference=w423, error in=w424, "Front Panel Window:Open"=TRUE) -> (reference out=w426:refnum<vi>, error out=w427:errorcluster)
                n179 = call-by-ref "?"(reference=w426, error in=w427, "Mode"=T44."Get Channel Names") -> (reference out=w428:refnum<vi>, error out=w429:errorcluster)  [unwired: 5 in]
                n180 = Close Reference(reference=w428, error in (no error)=w429) -> ()  [unwired: 1 out]
                n181 = event-data() -> ()  [unwired: 1 in, 5 out]
              }
              event "EnFlo Tun Display": Mouse Down? {
                n182 = event-data() -> ()  [unwired: 9 out]
                n183 = global read "Constants_global.vi" "EnFlo SW Folder"() -> (w443:path)
                n184 = Build Path(base path=w443, name or relative path=path "Anemometry/Utilities/EnFlo_Tunnel_Display.vi") -> (appended path=w438:path)
                n185 = Open VI Reference(vi path=w438) -> (vi reference=w437:refnum<vi>, error out=w436:errorcluster)  [unwired: 5 in]
                n186 = invoke class="VI" method="FP.Open"(reference=w437, error in=w436, "Activate"=TRUE ("Activate?"), "State"=T45."Standard") -> (reference out=w435:refnum<vi>, error out=w434:errorcluster)  [unwired: 1 in, 3 out]
                n187 = invoke class="VI" method="Run VI"(reference=w435, error in=w434, "Wait until done"=FALSE ("Wait Until Done"), "Auto Dispose Ref"=FALSE ("Wait until done")) -> (reference out=w439:refnum<vi>, error out=w440:errorcluster)  [unwired: 1 in, 3 out]
                n188 = Close Reference(reference=w439, error in (no error)=w440) -> ()  [unwired: 1 out]
                n189 = event-data() -> ()  [unwired: 5 in, 1 out]
              }
              event Mouse Down? {
                n190 = event-data() -> ()  [unwired: 5 out]
                n191 = global read "Constants_global.vi" "EnFlo SW Folder"() -> (w445:path)
                n192 = Build Path(base path=w445, name or relative path=path "ADAM Client/ADAM client VIs/Set_Tunnel_Speed.vi") -> (appended path=w448:path)
                n193 = call "Open_Close_Front_Panel.ph.vi"("Front Panel Window:Open"=TRUE, "VI path"=w448) -> ()  [unwired: 2 out]
                n194 = event-data() -> ()  [unwired: 1 in, 5 out]
              }
              event Mouse Down? {
                n195 = event-data() -> ()  [unwired: 5 out]
                n196 = global read "Constants_global.vi" "EnFlo SW Folder"() -> (w449:path)
                n197 = Build Path(base path=w449, name or relative path=path "ADAM Client/ADAM client VIs/Plot_Server_Data.vi") -> (appended path=w452:path)
                n198 = Open VI Reference(vi path=w452) -> (vi reference=w454:refnum<vi>, error out=w451:errorcluster)  [unwired: 1 in, 4 out]
                n199 = property class="VI"(reference=w454, error in=w451, "Front Panel Window:Open"=TRUE) -> (reference out=w455:refnum<vi>, error out=w456:errorcluster)
                n200 = invoke class="VI" method="Run VI"(reference=w455, error in=w456, "Wait until done"=FALSE, "Auto Dispose Ref"=TRUE) -> (reference out=w457:refnum<vi>, error out=w458:errorcluster)  [unwired: 1 in, 3 out]
                n201 = Close Reference(reference=w457, error in (no error)=w458) -> ()  [unwired: 1 out]
                n202 = event-data() -> ()  [unwired: 1 in, 5 out]
              }
              event Mouse Down? {
                n203 = event-data() -> ()  [unwired: 5 out]
                n204 = global read "Constants_global.vi" "EnFlo SW Folder"() -> (w468:path)
                n205 = Build Path(base path=w468, name or relative path=path "ADAM Server/ADAM_scan_table.vi") -> (appended path=w466:path)
                n206 = Open VI Reference(vi path=w466) -> (vi reference=w469:refnum<vi>, error out=w470:errorcluster)  [unwired: 1 in, 4 out]
                n207 = property class="VI"(reference=w469, error in=w470) -> (reference out=w464:refnum<vi>, error out=w463:errorcluster, "Execution:State"=w471:T46)
                n208 = Equal?(x=w471, y=T46."Run top level" ("Execution:State")) -> (x = y?=w465:bool)
                n209 = case shown="False" w465 {
                  tunnel: w464 -> [w476 w493]
                  tunnel: w463 -> [w475 w492]
                  tunnel: [w474 w493] -> w462
                  tunnel: [w473 w492] -> w461
                  frame False {
                    n210 = Two Button Dialog(message="Are you sure that you want to Run the ADAM Scan table on this machine?", 1:"Run" ("F button name (\"Cancel\")"), 2:"Cancel" ("T button name (\"OK\")")) -> (T button?=w477:bool)
                    n211 = case shown="False" w477 {
                      tunnel: w476 -> [w484 w491]
                      tunnel: w475 -> [w483 w490]
                      tunnel: [w482 w491] -> w474
                      tunnel: [w481 w490] -> w473
                      frame False {
                        n212 = property class="VI"(reference=w484, error in=w483, "Front Panel Window:Open"=TRUE) -> (reference out=w488:refnum<vi>, error out=w487:errorcluster)
                        n213 = invoke class="VI" method="Run VI"(reference=w488, error in=w487, "Wait until done"=FALSE, "Auto Dispose Ref"=TRUE) -> (reference out=w482:refnum<vi>, error out=w481:errorcluster)  [unwired: 1 in, 3 out]
                      }
                      frame True {
                      }
                    }
                  }
                  frame True {
                  }
                }
                n214 = event-data() -> ()  [unwired: 1 in, 2 out]
                n215 = Close Reference(reference=w462, error in (no error)=w461) -> ()  [unwired: 1 out]
              }
              event Mouse Down? {
                n216 = event-data() -> ()  [unwired: 5 out]
                n217 = global read "Constants_global.vi" "EnFlo SW Folder"() -> (w496:path)
                n218 = Build Path(base path=w496, name or relative path=path "ADAM Serial/Instrument drivers/Traverses/~subVIs/Read_Write_Trav_Config.vi") -> (appended path=w497:path)
                n219 = Build Path(base path=w496, name or relative path=path "ADAM Serial/Instrument drivers/Traverses/~subVIs/DriveConfigGlobal.vi") -> (appended path=w498:path)
                n220 = flat-sequence {
                  tunnel: w498 -> [w499]
                  tunnel: w497 -> [w501]
                  frame #0 {
                    n221 = call "Open_Close_Front_Panel.ph.vi"("Front Panel Window:Open"=TRUE, "VI path"=w499) -> ()  [unwired: 2 out]
                  }
                  frame #1 {
                    n222 = call "Open_Close_Front_Panel.ph.vi"("Front Panel Window:Open"=TRUE, "VI path"=w501) -> ()  [unwired: 2 out]
                  }
                }
                n223 = event-data() -> ()  [unwired: 1 in, 5 out]
              }
              event Mouse Down? {
                n224 = event-data() -> ()  [unwired: 5 out]
                n225 = global read "Constants_global.vi" "EnFlo SW Folder"() -> (w503:path)
                n226 = Build Path(base path=w503, name or relative path=path "Anemometry/Utilities/Hot_wire_Calculator.vi") -> (appended path=w506:path)
                n227 = call "Open_Close_Front_Panel.ph.vi"("Front Panel Window:Open"=TRUE, "VI path"=w506) -> ()  [unwired: 2 out]
                n228 = event-data() -> ()  [unwired: 1 in, 5 out]
              }
              event "Show Manual Sync": Mouse Down {
                n229 = event-data() -> ()  [unwired: 9 out]
                n230 = global read "Constants_global.vi" "EnFlo SW Folder"() -> (w507:path)
                n231 = Build Path(base path=w507, name or relative path=path "Anemometry/Utilities/EnFlo_Data_Sync_Manual.vi") -> (appended path=w510:path)
                n232 = call "Open_Close_Front_Panel.ph.vi"("Front Panel Window:Open"=TRUE, "VI path"=w510) -> ()  [unwired: 2 out]
              }
              event "Plot_FFID_Calibs.vi": Mouse Down {
                n233 = event-data() -> ()  [unwired: 9 out]
                n234 = global read "Constants_global.vi" "EnFlo SW Folder"() -> (w521:path)
                n235 = Build Path(base path=w521, name or relative path=path "ADAM Client/ADAM client VIs/Plot_FFID_Calibs.vi") -> (appended path=w511:path)
                n236 = Open VI Reference(vi path=w511) -> (vi reference=w514:refnum<vi>, error out=w512:errorcluster)  [unwired: 1 in, 4 out]
                n237 = property class="VI"(reference=w514, error in=w512, "Front Panel Window:Open"=TRUE) -> (reference out=w515:refnum<vi>, error out=w516:errorcluster)
                n238 = invoke class="VI" method="Run VI"(reference=w515, error in=w516, "Wait until done"=FALSE, "Auto Dispose Ref"=TRUE) -> (reference out=w517:refnum<vi>, error out=w518:errorcluster)  [unwired: 1 in, 3 out]
                n239 = Close Reference(reference=w517, error in (no error)=w518) -> ()  [unwired: 1 out]
              }
              event "Beam Check Positions": Mouse Down {
                n240 = event-data() -> ()  [unwired: 9 out]
                n241 = global read "Constants_global.vi" "EnFlo SW Folder"() -> (w533:path)
                n242 = Build Path(base path=w533, name or relative path=path "Anemometry/Anemometry Sub Vis/LDA/Beam_Check_Positions.vi") -> (appended path=w524:path)
                n243 = Open VI Reference(type specifier VI Refnum (for type only)=refnum<vi> refnum, vi path=w524) -> (vi reference=w526:refnum<vi>, error out=w527:errorcluster)  [unwired: 1 in, 3 out]
                n244 = property class="VI Interface Type 3"(reference=w526, error in=w527, "Front Panel Window:Open"=TRUE) -> (reference out=w529:refnum<vi>, error out=w530:errorcluster)
                n245 = call-by-ref "?"(reference=w529, error in=w530, "Mode"=T47."Load From Excel File") -> (reference out=w531:refnum<vi>, error out=w532:errorcluster)  [unwired: 2 in, 1 out]
                n246 = Close Reference(reference=w531, error in (no error)=w532) -> ()  [unwired: 1 out]
              }
              event Mouse Down? {
                n247 = event-data() -> ()  [unwired: 5 out]
                n248 = global read "Constants_global.vi" "EnFlo SW Folder"() -> (w535:path)
                n249 = Build Path(base path=w535, name or relative path=path "Anemometry/Utilities/Hydrosonic_Manual.vi") -> (appended path=w538:path)
                n250 = call "Open_Close_Front_Panel.ph.vi"("Front Panel Window:Open"=TRUE, "VI path"=w538) -> ()  [unwired: 2 out]
                n251 = event-data() -> ()  [unwired: 1 in, 5 out]
              }
              event "Top Level Traverse": Mouse Down {
                n252 = event-data() -> ()  [unwired: 9 out]
                n253 = global read "Constants_global.vi" "EnFlo SW Folder"() -> (w539:path)
                n254 = Build Path(base path=w539, name or relative path=path "Anemometry/Utilities/Top_Level_Move_Traverse.vi") -> (appended path=w542:path)
                n255 = call "Open_Close_Front_Panel.ph.vi"("Front Panel Window:Open"=TRUE, "VI path"=w542) -> ()  [unwired: 2 out]
              }
              event "Post_Pro_Results_Hierarchy": Mouse Down {
                n256 = event-data() -> ()  [unwired: 9 out]
                n257 = global read "Constants_global.vi" "EnFlo SW Folder"() -> (w543:path)
                n258 = Build Path(base path=w543, name or relative path=path "Anemometry/Utilities/Post_Pro_Results_Hierarchy.vi") -> (appended path=w546:path)
                n259 = call "Open_Close_Front_Panel.ph.vi"("Front Panel Window:Open"=TRUE, "VI path"=w546) -> ()  [unwired: 2 out]
              }
              event Mouse Down? {
                n260 = event-data() -> ()  [unwired: 5 out]
                n261 = global read "Constants_global.vi" "EnFlo SW Folder"() -> (w547:path)
                n262 = Build Path(base path=w547, name or relative path=path "ADAM Client/ADAM client VIs/Fast_FID_Valve_Control.vi") -> (appended path=w550:path)
                n263 = call "Open_Close_Front_Panel.ph.vi"("Front Panel Window:Open"=TRUE, "VI path"=w550) -> ()  [unwired: 2 out]
                n264 = event-data() -> ()  [unwired: 1 in, 5 out]
              }
              event Mouse Down? {
                n265 = event-data() -> ()  [unwired: 5 out]
                n266 = global read "Constants_global.vi" "EnFlo SW Folder"() -> (w551:path)
                n267 = Build Path(base path=w551, name or relative path=path "Anemometry/Utilities/Preference_Panel.vi") -> (appended path=w560:path)
                n268 = Open VI Reference(type specifier VI Refnum (for type only)=refnum<vi> refnum, vi path=w560) -> (vi reference=w553:refnum<vi>, error out=w554:errorcluster)  [unwired: 1 in, 3 out]
                n269 = property class="VI Interface Type 4"(reference=w553, error in=w554, "Front Panel Window:Open"=TRUE) -> (reference out=w556:refnum<vi>, error out=w557:errorcluster)
                n270 = call-by-ref "?"(reference=w556, error in=w557, "Mode"=Preference_Mode."Load, Edit then Save") -> (reference out=w558:refnum<vi>, error out=w559:errorcluster)
                n271 = Close Reference(reference=w558, error in (no error)=w559) -> ()  [unwired: 1 out]
                n272 = event-data("Discard?"=TRUE) -> ()  [unwired: 1 in, 4 out]
              }
              event Mouse Down? {
                n273 = event-data() -> ()  [unwired: 5 out]
                n274 = global read "Constants_global.vi" "EnFlo SW Folder"() -> (w567:path)
                n275 = Build Path(base path=w567, name or relative path=path "ADAM Client/Sub VIs/Gas_Setup.vi") -> (appended path=w574:path)
                n276 = Open VI Reference(type specifier VI Refnum (for type only)=refnum<vi> refnum, vi path=w574) -> (vi reference=w570:refnum<vi>, error out=w571:errorcluster)  [unwired: 1 in, 3 out]
                n277 = property class="VI Interface Type 5"(reference=w570, error in=w571, "Front Panel Window:Open"=TRUE) -> (reference out=w575:refnum<vi>, error out=w573:errorcluster)
                n278 = call-by-ref "?"(reference=w575, error in=w573) -> (reference out=w565:refnum<vi>, error out=w564:errorcluster)  [unwired: 9 in]
                n279 = Close Reference(reference=w565, error in (no error)=w564) -> ()  [unwired: 1 out]
                n280 = event-data("Discard?"=TRUE) -> ()  [unwired: 1 in, 4 out]
              }
              event Mouse Down? {
                n281 = event-data() -> ()  [unwired: 5 out]
                n282 = global read "Constants_global.vi" "EnFlo SW Folder"() -> (w579:path)
                n283 = Build Path(base path=w579, name or relative path=path "ADAM Client/Sub VIs/User_Metadata.vi") -> (appended path=w586:path)
                n284 = Open VI Reference(type specifier VI Refnum (for type only)=refnum<vi> refnum, vi path=w586) -> (vi reference=w582:refnum<vi>, error out=w583:errorcluster)  [unwired: 1 in, 3 out]
                n285 = property class="VI Interface Type 5"(reference=w582, error in=w583, "Front Panel Window:Open"=TRUE) -> (reference out=w587:refnum<vi>, error out=w585:errorcluster)
                n286 = call-by-ref "?"(reference=w587, error in=w585) -> (reference out=w577:refnum<vi>, error out=w576:errorcluster)  [unwired: 9 in]
                n287 = Close Reference(reference=w577, error in (no error)=w576) -> ()  [unwired: 1 out]
                n288 = event-data("Discard?"=TRUE) -> ()  [unwired: 1 in, 4 out]
              }
              event Mouse Down? {
                n289 = event-data() -> ()  [unwired: 5 out]
                n290 = global read "Constants_global.vi" "EnFlo SW Folder"() -> (w593:path)
                n291 = Build Path(base path=w593, name or relative path=path "ADAM Client/Sub VIs/EnFlo_Tunnel_Setup.vi") -> (appended path=w596:path)
                n292 = Open VI Reference(type specifier VI Refnum (for type only)=refnum<vi> refnum, vi path=w596) -> (vi reference=w590:refnum<vi>, error out=w589:errorcluster)  [unwired: 1 in, 3 out]
                n293 = call-by-ref "?"(reference=w590, error in=w589) -> (reference out=w592:refnum<vi>, error out=w591:errorcluster)  [unwired: 9 in]
                n294 = Close Reference(reference=w592, error in (no error)=w591) -> ()  [unwired: 1 out]
                n295 = event-data("Discard?"=TRUE) -> ()  [unwired: 1 in, 4 out]
              }
              event Mouse Down? {
                w610 = TRUE  # Show Panel?
                n296 = event-data() -> ()  [unwired: 5 out]
                n297 = global read "Preference_global.vi" "Use New Collision Code"() -> (w600:bool)
                n298 = global read "Constants_global.vi" "EnFlo SW Folder"() -> (w606:path)
                n299 = Select(t=path "Anemometry/Anemometry Sub Vis/Gen Trav/Traverse_Space_for new collision code.vi", s=w600, f=path "Anemometry/Anemometry Sub Vis/Gen Trav/Traverse_Space.vi") -> (s? t:f=w597:path)
                n300 = Build Path(base path=w606, name or relative path=w597) -> (appended path=w608:path)
                n301 = global read "Trav_pos_global.vi" "Default Traverse Setup"() -> (w601:string)
                n302 = Open VI Reference(type specifier VI Refnum (for type only)=refnum<vi> refnum, vi path=w608) -> (vi reference=w609:refnum<vi>, error out=w602:errorcluster)  [unwired: 1 in, 3 out]
                n303 = call-by-ref "?"(reference=w609, error in=w602, "Show Panel?"=w610, "Traverse Setup"=w601) -> (reference out=w604:refnum<vi>, error out=w603:errorcluster)  [unwired: 8 in, 1 out]
                n304 = Close Reference(reference=w604, error in (no error)=w603) -> ()  [unwired: 1 out]
                n305 = event-data("Discard?"=TRUE) -> ()  [unwired: 1 in, 4 out]
              }
              event Mouse Down? {
                n306 = event-data() -> ()  [unwired: 5 out]
                n307 = global read "Constants_global.vi" "EnFlo SW Folder"() -> (w612:path)
                n308 = Build Path(base path=w612, name or relative path=path "Anemometry/Anemometry Sub Vis/Traverse vi's/EnFlo Tunnel specific/Check_EnFlo_Arm.vi") -> (appended path=w614:path)
                n309 = call "Open_Close_Front_Panel.ph.vi"("Front Panel Window:Open"=TRUE, "VI path"=w614) -> ()  [unwired: 2 out]
                n310 = event-data() -> ()  [unwired: 1 in, 2 out]
              }
              event Mouse Down? {
                n311 = event-data() -> ()  [unwired: 5 out]
                n312 = global read "Constants_global.vi" "EnFlo SW Folder"() -> (w622:path)
                n313 = Build Path(base path=w622, name or relative path=path "Anemometry/Anemometry Sub Vis/Gen Trav/3D_Traverse_move.vi") -> (appended path=w619:path)
                n314 = Strip Path(path=w619) -> (name=w618:string)  [unwired: 1 out]
                n315 = Open VI Reference(vi path=w618) -> (vi reference=w620:refnum<vi>, error out=w621:errorcluster)  [unwired: 1 in, 4 out]
                n316 = property class="VI"(reference=w620, error in=w621) -> (reference out=w616:refnum<vi>, error out=w615:errorcluster, "Front Panel Window:Open"=w617:bool)
                n317 = case shown="False" w617 {
                  tunnel: w619 -> [w625 _]
                  tunnel: w616 -> [_ w642]
                  tunnel: w615 -> [_ w641]
                  frame False {
                    w624 = TRUE  # Last Part of Move?
                    n318 = global read "Trav_pos_global.vi" "Work in Tunnel Coordinates?"() -> (w635:T54)
                    n319 = global read "Trav_pos_global.vi" "Default Traverse Setup"() -> (w633:string)
                    n320 = Open VI Reference(type specifier VI Refnum (for type only)=refnum<vi> refnum, vi path=w625) -> (vi reference=w629:refnum<vi>, error out=w630:errorcluster)  [unwired: 1 in, 3 out]
                    n321 = property class="VI Interface Type 6"(reference=w629, error in=w630, "Front Panel Window:Open"=TRUE) -> (reference out=w626:refnum<vi>, error out=w627:errorcluster)
                    n322 = call-by-ref "?"(reference=w626, error in=w627, "Mode"=Trav_mode."Read traverse position", "Work in Tunnel Coordinates"=w635, "Simulate/Run"=User_Specific_mode."Run VI", "Traverse name"=w633, "Last Part of Move?"=w624) -> (reference out=w631:refnum<vi>, error out=w632:errorcluster)  [unwired: 12 in, 3 out]
                    n323 = Close Reference(reference=w631, error in (no error)=w632) -> ()  [unwired: 1 out]
                  }
                  frame True {
                    n324 = property class="VI"(reference=w642, error in=w641, "Front Panel Window:Open"=TRUE) -> (reference out=w640:refnum<vi>, error out=w639:errorcluster)
                    n325 = Close Reference(reference=w640, error in (no error)=w639) -> ()  [unwired: 1 out]
                  }
                }
                n326 = event-data() -> ()  [unwired: 1 in, 5 out]
              }
              event Mouse Down? {
                n327 = event-data() -> ()  [unwired: 5 out]
                n328 = Open VI Reference(vi path="Multi_Run_Prog.vi") -> (vi reference=w648:refnum<vi>, error out=w647:errorcluster)  [unwired: 1 in, 4 out]
                n329 = property class="VI"(reference=w648, error in=w647, "Front Panel Window:Open"=TRUE) -> (reference out=w645:refnum<vi>, error out=w646:errorcluster)
                n330 = Close Reference(reference=w645, error in (no error)=w646) -> (error out=w643:errorcluster)
                n331 = Unbundle By Name(w643) -> ("status"=w650:bool)
                n332 = case shown="True" w650 {
                  frame False {
                  }
                  frame True {
                    n333 = global read "Constants_global.vi" "EnFlo SW Folder"() -> (w658:path)
                    n334 = call "Setup_Filepath.vi"("Setup File Type"=Setup_Filetype."General", "Filename in"="Multi_Run_Filename.txt" ("name or relative path")) -> ("Filename Out"=w651:path)  [unwired: 1 out]
                    n335 = Build Path(base path=w658, name or relative path=path "Anemometry/Multi_Run_Prog.vi") -> (appended path=w657:path)
                    n336 = call "Read_File_Simple.vi"("Filename"=w651) -> ("string"=w656:string)  [unwired: 2 in, 7 out]
                    n337 = String To Path(string=w656) -> (path=w654:path)
                    n338 = call "Does_file_exist_(simple).vi"("Pathname"=w654) -> ("exists?"=w655:bool)
                    n339 = case shown="True" w655 {
                      tunnel: w657 -> [w660 w672]
                      tunnel: w654 -> [_ w670]
                      frame False {
                        n340 = call "Open_Close_Front_Panel.ph.vi"("Front Panel Window:Open"=TRUE, "VI path"=w660) -> ()  [unwired: 2 out]
                      }
                      frame True {
                        n341 = Open VI Reference(type specifier VI Refnum (for type only)=refnum<vi> refnum, vi path=w672) -> (vi reference=w669:refnum<vi>, error out=w668:errorcluster)  [unwired: 1 in, 3 out]
                        n342 = property class="VI Interface Type 8"(reference=w669, error in=w668, "Front Panel Window:Open"=TRUE) -> (reference out=w666:refnum<vi>, error out=w667:errorcluster)
                        n343 = call-by-ref "?"(reference=w666, error in=w667, "Command filename"=w670, "Mode"=T51."Load Command File" ("Setup mode")) -> (reference out=w665:refnum<vi>, error out=w664:errorcluster)  [unwired: 18 in]
                        n344 = Close Reference(reference=w665, error in (no error)=w664) -> ()  [unwired: 1 out]
                      }
                    }
                  }
                }
                n345 = event-data() -> ()  [unwired: 1 in, 5 out]
              }
              event Mouse Down? {
                w674 = "Calibration.vi" ("name or relative path")
                n346 = event-data() -> ()  [unwired: 5 out]
                n347 = global read "Constants_global.vi" "EnFlo SW Folder"() -> (w680:path)
                n348 = Open VI Reference(vi path=w674) -> (vi reference=w678:refnum<vi>, error out=w677:errorcluster)  [unwired: 1 in, 4 out]
                n349 = Build Path(base path=w680, name or relative path="Anemometry") -> (appended path=w683:path)
                n350 = property class="VI"(reference=w678, error in=w677, "Front Panel Window:Open"=TRUE) -> (reference out=w675:refnum<vi>, error out=w676:errorcluster)
                n351 = Build Path(base path=w683, name or relative path=w674) -> (appended path=w681:path)
                n352 = Close Reference(reference=w675, error in (no error)=w676) -> (error out=w673:errorcluster)
                n353 = Unbundle By Name(w673) -> ("status"=w682:bool)
                n354 = case shown="True" w682 {
                  tunnel: w681 -> [_ w685]
                  tunnel: w673 -> [_ _]
                  frame False {
                  }
                  frame True {
                    n355 = stacked-sequence {
                      seq-local: [w691 _] -> [_ w698]
                      tunnel: w685 -> [_ w699]
                      frame #0 {
                        n356 = call "Setup_Filepath.vi"("Setup File Type"=Setup_Filetype."Calibration Setups", "Filename in"="Current_Setup.xls") -> ("Filename Out"=w686:path)  [unwired: 1 out]
                        n357 = call "Read_File_Simple.vi"("Filename"=w686) -> ("string"=w695:string)  [unwired: 2 in, 7 out]
                        n358 = Format Into String(format string="Calibration Setup File   %s", w686) -> (resulting string=w689:string)  [unwired: 2 in, 1 out]
                        n359 = call "Get_string_subset.vi"("String Name"=w689, "String to split"=w695, "File Label"="Raw data header") -> ("Output string"=w693:string)  [unwired: 1 in, 1 out]
                        n360 = call "Get_Characters_from_string.vi"("Input string"=w693, "Variable name"="Calib filename") -> ("Value"=w692:string)  [unwired: 1 in, 1 out]
                        n361 = call "String_to_Pathname.vi"("Input String"=w692) -> ("path"=w691:path)
                      }
                      frame #1 {
                        n362 = call "Does_file_exist_(simple).vi"("Pathname"=w698) -> ("exists?"=w697:bool)
                        n363 = case shown="True" w697 {
                          tunnel: w699 -> [w700 w715]
                          tunnel: w698 -> [_ w709]
                          frame False {
                            n364 = call "Open_Close_Front_Panel.ph.vi"("Front Panel Window:Open"=TRUE, "VI path"=w700) -> ()  [unwired: 2 out]
                          }
                          frame True {
                            w707 = TRUE ("Front Panel Window:Open")
                            n365 = Open VI Reference(type specifier VI Refnum (for type only)=refnum<vi> refnum, vi path=w715) -> (vi reference=w713:refnum<vi>, error out=w708:errorcluster)  [unwired: 1 in, 3 out]
                            n366 = property class="VI Interface Type 7"(reference=w713, error in=w708, "Front Panel Window:Open"=w707, "Front Panel Window:Auto Center (Deprecated)"=w707) -> (reference out=w712:refnum<vi>, error out=w711:errorcluster)
                            n367 = call-by-ref "?"(reference=w712, error in=w711, "Mode"=Calib_mode."Setup Front Panel", "Calib file"=w709) -> (reference out=w705:refnum<vi>, error out=w704:errorcluster)  [unwired: 15 in, 3 out]
                            n368 = property class="VI Interface Type 7"(reference=w705, error in=w704, "Front Panel Window:Auto Center (Deprecated)"=FALSE ("Front Panel Window:Auto Center")) -> (reference out=w703:refnum<vi>, error out=w702:errorcluster)
                            n369 = Close Reference(reference=w703, error in (no error)=w702) -> ()  [unwired: 1 out]
                          }
                        }
                      }
                    }
                  }
                }
                n370 = event-data() -> ()  [unwired: 1 in, 5 out]
              }
              event "stop": Mouse Down? {
                n371 = event-data() -> ()  [unwired: 5 out]
                n372 = flat-sequence {
                  frame #0 {
                    n373 = global write "Dynamic_call_global.ph.vi" "EnFlo Hub running?"(FALSE ("EnFlo Hub running?")) -> ()
                  }
                  frame #1 {
                    n374 = Stop(stop? (T)=TRUE) -> ()
                  }
                }
                n375 = event-data() -> ()  [unwired: 1 in, 4 out]
              }
              event "Rig_Control": Value Change {
                n376 = event-data() -> ("OldVal"=w719:cluster{"Ch Name":string, "Boolean":bool}[], "NewVal"=w718:cluster{"Ch Name":string, "Boolean":bool}[])  [unwired: 5 out]
                n377 = for {
                  tunnel: w719 -> [w725] mode=indexing
                  tunnel: w718 -> [w724] mode=indexing
                  n378 = Unbundle By Name(w725) -> ("Ch Name"=w722:string, "Boolean"=w723:bool)
                  n379 = Unbundle By Name(w724) -> ("Boolean"=w721:bool)  [unwired: 1 out]
                  n380 = Not Equal?(x=w723, y=w721) -> (x != y?=w720:bool)
                  n381 = case shown="True" w720 {
                    tunnel: w722 -> [_ w729]
                    tunnel: w721 -> [_ w726]
                    frame False {
                    }
                    frame True {
                      n382 = case shown="False" w726 {
                        tunnel: ["Off" "On"] -> w728
                        tunnel: [0.0 ("f") 1.0 ("t")] -> w727
                        frame False {
                        }
                        frame True {
                        }
                      }
                      n383 = Format Into String(format string="Are you sure you want to turn %s %s?", w729, w728) -> (resulting string=w734:string)  [unwired: 2 in, 1 out]
                      n384 = Format Into String(format string="Make  %s  %s", w729, w728) -> (resulting string=w730:string)  [unwired: 2 in, 1 out]
                      n385 = Two Button Dialog(message=w734, 1:w730, 2:"Cancel" ("T button name (\"OK\")")) -> (T button?=w732:bool)
                      n386 = case shown="False" w732 {
                        tunnel: w729 -> [w741 _]
                        tunnel: w727 -> [w740 _]
                        frame False {
                          n387 = Build Array(w740) -> (w743:dbl[])
                          n388 = Build Array(w741) -> (w742:string[])
                          n389 = call "ASYNC_Adam_client.vi"("Values"=w743, "Channel Names"=w742) -> ()  [unwired: 1 in, 2 out]
                        }
                        frame True {
                        }
                      }
                    }
                  }
                }
              }
            }
          }
        }
        "Numeric" <- w272
      }
      n390 = while {
        shift-left: _ -> [w746]
        shift-right: [w747] -> _
        shift-left: "Initialise" -> [w745]
        shift-right: [w748] -> _
        i -> [w744]
        stop <- TRUE continue-if-true
        n391 = case shown="\"Initialise\"" w745 {
          tunnel: ["End" "Initialise" "Wait for call remote sub vi occurrence" "Check type of VI to launch" w775 "Wait until remote sub vi is opened" "Update opened vis array" "Update opened vis array" "Update opened vis array" "Wait until remote sub vi is opened" "Wait for call remote sub vi occurrence"] -> w748
          tunnel: [w750 w763 w766 errorcluster {"status"=FALSE, "code"=0, "source"=""} ("error out") w771 w786 w816 w833 w848 w888 w908] -> w747
          tunnel: w746 -> [w750 w763 w766 _ w771 w786 _ _ _ w888 w908]
          tunnel: w745 -> [w752 _ _ _ _ _ _ _ _ _ _]
          tunnel: w744 -> [_ _ _ _ _ _ _ _ _ _ _]
          frame "No match", Default {
            n392 = Current VI's Path() -> (path=w753:path)
            n393 = Format Into String(format string="The Case\"%s\" was not Matched\nin VI named\n'%s\"" ("Format String"), w752, w753) -> (resulting string=w756:string)  [unwired: 2 in, 1 out]
            n394 = One Button Dialog(message=w756, button name ("OK")="STOP") -> (true=w754:bool)
            n395 = Stop(stop? (T)=w754) -> ()
          }
          frame "Never run" {
            # "This keeps the Coherent global and DLL reference alive even after all associated vi's are closed and the Hub is stopped (but not closed, that really is game over....)"
            # "These globals are here to make sure they stay in memory\nafter \"Preference Panel\" has finished running"
            n396 = call "Email_With_Log.vi"() -> ()  [unwired: 4 in, 3 out]
            n397 = call "Remember_value.vi"() -> ()  [unwired: 3 in, 1 out]
            n398 = call "Output_Trav_Pos.vi"() -> ()  [unwired: 5 in, 1 out]
            n399 = call "Read_Write_Local_table.vi"() -> ()  [unwired: 3 in, 3 out]
            n400 = call "Overhead_Factor.vi"() -> ()  [unwired: 4 in, 1 out]
            n401 = global read "Trav_pos_global.vi" "Dummy Measurement?"() -> (→"Dummy Measurement":bool)
            n402 = global read "PWAtasksGLOBAL.vi" "Analogue Dev Name"() -> (→"Analogue Dev Name":string)
            n403 = global read "Constants_global.vi" "All_Users"() -> (→"All Users":path)
            n404 = global read "Preference_global.vi" "Rig Setup"() -> (→"Rig Name":string)
            n405 = call "Get DLL version.vi"() -> ()  [unwired: 3 out]
          }
          frame "Initialise" {
            "Iterations" <- 0 ("Iterations")
          }
          frame "Wait for call remote sub vi occurrence" {
            n406 = global read "Dynamic_call_global.ph.vi" "Call Remote Subvi"() -> (w769:refnum<k4>)
            n407 = Wait on Occurrence(2:w769) -> ()  [unwired: 3 out]
          }
          frame "Check type of VI to launch" {
            n408 = global read "Dynamic_call_global.ph.vi" "VI name to launch"() -> (w773:string)
            n409 = Match Pattern(string=w773, regular expression=";") -> (before substring=w770:string, after substring=w772:string)  [unwired: 3 out]
            n410 = case shown="\"Open LDA PWA & An\"" w770 {
              tunnel: ["Open vi" "Open application reference" "Open Analogue input server" w783] -> w775
              tunnel: [w778 w780 w782 w784] -> w774
              tunnel: w773 -> [w778 _ _ _]
              tunnel: w772 -> [_ w780 w782 w784]
              tunnel: w770 -> [_ _ _ w783]
              frame "Other", Default {
              }
              frame "Open Application Reference" {
              }
              frame "Open Analogue Input VI" {
              }
              frame "Open LDA PWA & An" {
              }
            }
            "VI Name" <- w774
          }
          frame "Open application reference" {
            n411 = local read "VI Name"() -> (w787:string)
            n412 = Match Pattern(string=w787, regular expression=";") -> (before substring=w795:string, after substring=w796:string)  [unwired: 3 out]
            n413 = Decimal String To Number(string=w796) -> (number=w797:i32)  [unwired: 3 out]
            n414 = To Unsigned Long Integer(number=w797) -> (unsigned 32bit integer=w794:u32)
            n415 = call "App_Ref_Global.vi"("Mode"=App_Global."Read Global") -> ("Output Array"=w793:T55[])  [unwired: 1 in, 1 out]
            n416 = Open Application Reference(10:w794, 11:w795) -> (0:w788:errorcluster, 3:w792:refnum<vi>)  [unwired: 1 in, 1 out]
            n417 = for {
              tunnel: w793 -> [w799] mode=indexing
              tunnel: w787 -> [w803]
              tunnel: w792 -> [w801]
              tunnel: [w800] -> w791 mode=indexing
              n418 = Unbundle By Name(w799) -> ("Server IP & Port No"=w804:string)
              n419 = Equal?(x=w804, y=w803) -> (x = y?=w802:bool)
              n420 = case shown="False" w802 {
                tunnel: w801 -> [_ w808]
                tunnel: [w805 w807] -> w800
                tunnel: w799 -> [w805 w806]
                frame False {
                }
                frame True {
                  n421 = Bundle By Name(cluster=w806, "Application reference"=w808) -> (w807:T55)
                }
              }
            }
            n422 = global write "Dynamic_call_global.ph.vi" "Error Cluster"(w788) -> ()
            n423 = call "App_Ref_Global.vi"("Input Array"=w791, "Mode"=App_Global."Write to Global") -> ()  [unwired: 2 out]
          }
          frame "Open Analogue input server" {
            n424 = local read "VI Name"() -> (w813:string)
            n425 = call "Get_link_info.vi"("VI Name"=w813) -> ("Path name"=w810:path, "Application reference"=w811:refnum<vi>, "Local Call?"=w812:bool)  [unwired: 1 out]
            n426 = global read "Dynamic_call_global.ph.vi" "Analogue Input"() -> (w815:refnum<vi>)
            n427 = case shown="True" w812 {
              tunnel: w815 -> [w821 w825]
              tunnel: [w817 w824] -> w814
              tunnel: [w820 w823] -> w816
              tunnel: w813 -> [w819 _]
              tunnel: w811 -> [w818 _]
              tunnel: w810 -> [_ w822]
              frame False {
                n428 = Open VI Reference(type specifier VI Refnum (for type only)=w821, application reference (local)=w818, vi path=w819) -> (vi reference=w817:refnum<vi>, error out=w820:errorcluster)  [unwired: 1 in, 2 out]
              }
              frame True {
                n429 = Open VI Reference(type specifier VI Refnum (for type only)=w825, vi path=w822) -> (vi reference=w824:refnum<vi>, error out=w823:errorcluster)  [unwired: 1 in, 3 out]
              }
            }
            n430 = global write "Dynamic_call_global.ph.vi" "Analogue Input"(w814) -> ()
          }
          frame "Open LDA PWA & An" {
            n431 = local read "VI Name"() -> (w830:string)
            n432 = call "Get_link_info.vi"("VI Name"=w830) -> ("Path name"=w827:path, "Application reference"=w828:refnum<vi>, "Local Call?"=w829:bool)  [unwired: 1 out]
            n433 = global read "Dynamic_call_global.ph.vi" "Take LDA PWA & An"() -> (w832:refnum<vi>)
            n434 = case shown="True" w829 {
              tunnel: w832 -> [w838 w842]
              tunnel: [w834 w841] -> w831
              tunnel: [w837 w840] -> w833
              tunnel: w830 -> [w836 _]
              tunnel: w828 -> [w835 _]
              tunnel: w827 -> [_ w839]
              frame False {
                n435 = Open VI Reference(type specifier VI Refnum (for type only)=w838, application reference (local)=w835, vi path=w836) -> (vi reference=w834:refnum<vi>, error out=w837:errorcluster)  [unwired: 1 in, 2 out]
              }
              frame True {
                n436 = Open VI Reference(type specifier VI Refnum (for type only)=w842, vi path=w839) -> (vi reference=w841:refnum<vi>, error out=w840:errorcluster)  [unwired: 1 in, 3 out]
              }
            }
            n437 = global write "Dynamic_call_global.ph.vi" "Take LDA PWA & An"(w831) -> ()
          }
          frame "Open vi" {
            n438 = local read "VI Name"() -> (w847:string)
            n439 = call "Get_link_info.vi"("VI Name"=w847) -> ("Path name"=w846:path, "Application reference"=w845:refnum<vi>, "Local Call?"=w844:bool)  [unwired: 1 out]
            n440 = case shown="\"No Match\", Default" w847 {
              tunnel: [w849 w858 w870] -> w848
              tunnel: w847 -> [w854 w857 w874]
              tunnel: w846 -> [_ _ w871]
              tunnel: w845 -> [_ w856 w873]
              tunnel: w844 -> [_ w855 w872]
              frame "No Match", Default {
                n441 = Format Into String(format string="VI named \"%s\" Not matched" ("Format String"), w854) -> (resulting string=w851:string)  [unwired: 2 in, 1 out]
                n442 = Bundle By Name(cluster=errorcluster {"status"=FALSE, "code"=0, "source"=""} ("error out"), "source"=w851, "status"=TRUE ("Bundle Element")) -> (w849:errorcluster)
              }
              frame "Program_Active_server.vi" {
                n443 = global read "Dynamic_call_global.ph.vi" "Program Active server"() -> (w860:refnum<vi>)
                n444 = case shown="True" w855 {
                  tunnel: w860 -> [w865 w869]
                  tunnel: [w864 w868] -> w859
                  tunnel: [w863 w867] -> w858
                  tunnel: w857 -> [w862 w866]
                  tunnel: w856 -> [w861 _]
                  frame False {
                    n445 = Open VI Reference(type specifier VI Refnum (for type only)=w865, application reference (local)=w861, vi path=w862) -> (vi reference=w864:refnum<vi>, error out=w863:errorcluster)  [unwired: 1 in, 2 out]
                  }
                  frame True {
                    n446 = Open VI Reference(type specifier VI Refnum (for type only)=w869, vi path=w866) -> (vi reference=w868:refnum<vi>, error out=w867:errorcluster)  [unwired: 1 in, 3 out]
                  }
                }
                n447 = global write "Dynamic_call_global.ph.vi" "Program Active server"(w859) -> ()
              }
              frame "GPIB_Server.vi" {
                n448 = global read "Dynamic_call_global.ph.vi" "GPIB_Server.vi"() -> (w876:refnum<vi>)
                n449 = case shown="False" w872 {
                  tunnel: w876 -> [w881 w885]
                  tunnel: [w880 w884] -> w875
                  tunnel: [w879 w883] -> w870
                  tunnel: w874 -> [w877 _]
                  tunnel: w873 -> [w878 _]
                  tunnel: w871 -> [_ w882]
                  frame False {
                    n450 = Open VI Reference(type specifier VI Refnum (for type only)=w881, application reference (local)=w878, vi path=w877) -> (vi reference=w880:refnum<vi>, error out=w879:errorcluster)  [unwired: 1 in, 2 out]
                  }
                  frame True {
                    n451 = Open VI Reference(type specifier VI Refnum (for type only)=w885, vi path=w882) -> (vi reference=w884:refnum<vi>, error out=w883:errorcluster)  [unwired: 1 in, 3 out]
                  }
                }
                n452 = global write "Dynamic_call_global.ph.vi" "GPIB_Server.vi"(w875) -> ()
              }
            }
          }
          frame "Update opened vis array" {
            w890 = TRUE  # Dialog Box
            n453 = local read "VI Name"() -> (w889:string)
            n454 = Unbundle By Name(w888) -> ("status"=w893:bool, "source"=w891:string)
            n455 = case shown="True" w893 {
              tunnel: w888 -> [w895 w904]
              tunnel: [w895 w903] -> w892
              tunnel: w889 -> [w896 w899]
              tunnel: w891 -> [_ w902]
              frame False {
                n456 = global read "Dynamic_call_global.ph.vi" "Opened VIs"() -> (w897:string[])
                n457 = To Upper Case(1:w896) -> (0:w894:string)
                n458 = Build Array (concatenate)(w897, w894) -> (w898:string[])
                n459 = global write "Dynamic_call_global.ph.vi" "Opened VIs"(w898) -> ()
              }
              frame True {
                n460 = Concatenate Strings(w899, " " ("Substring"), w902) -> (w900:string)
                n461 = Bundle By Name(cluster=w904, "source"=w900) -> (w903:errorcluster)
              }
            }
            n462 = call "EnFlo_Error_Handler.vi"("error in (no error)"=w892, "Error Type"="Dynamic Call", "Dialog Box (T)"=w890) -> ()  [unwired: 3 out]
          }
          frame "Wait until remote sub vi is opened" {
            n463 = global read "Dynamic_call_global.ph.vi" "Remote Subvi Opened"() -> (w909:refnum<k4>)
            n464 = local read "Iterations"() -> (w907:i32)
            n465 = Increment(x=w907) -> (x+1=w906:i32)
            n466 = local write "Iterations"(w906) -> ()
            n467 = Set Occurrence(w909) -> ()
          }
        }
      }
      n468 = while {
        i -> [w45]
        stop <- FALSE stop-if-true
        n469 = stacked-sequence {
          tunnel: w45 -> [_ w93 w101]
          frame #0 {
            n470 = global read "Dynamic_call_global.ph.vi" "EnFlo Hub running?"() -> (w49:bool)
            n471 = Equal?(x="Tab Control", y=T40."Adam Table" ("Tab Control")) -> (x = y?=w50:bool)
            n472 = And(x=w50, y=w49) -> (x .and. y?=w48:bool)
            n473 = case shown="True" w48 {
              frame True {
                n474 = local read "List of ADAM channels to view"() -> (w59:string[])
                n475 = local read "List of ADAM control channels"() -> (w62:string[])
                n476 = Build Array (concatenate)(w62, w59) -> (w61:string[])
                n477 = call "Get_Current_Scan_client.vi"("ADAM Ch Names"=w61) -> ("Ch Description Array"=w56:T56[], "Numerical Values"=w60:dbl[])  [unwired: 2 out]
                n478 = Array Size(array=w62) -> (size(s)=w57:i32)
                n479 = Array Subset(array=w56, index=w57) -> (w55:T56[])  [unwired: 1 in]
                n480 = Array Subset(array=w60, index=w57) -> (w54:dbl[])  [unwired: 1 in]
                n481 = for {
                  tunnel: w55 -> [w69] mode=indexing
                  tunnel: [w68] -> w53 mode=indexing
                  tunnel: cluster{"Ch Name":string, "Numeric":dbl} {"Ch Name"="", "Numeric"=0.0} ("Cluster") -> [w67]
                  tunnel: w54 -> [w65] mode=indexing
                  n482 = Unbundle By Name(w69) -> ("Ch Name"=w66:string)
                  n483 = Bundle By Name(cluster=w67, "Ch Name"=w66, "Numeric"=w65) -> (w68:cluster{"Ch Name":string, "Numeric":dbl})
                }
                "Current Values" <- w53
                n484 = for {
                  N: w57 -> [_]
                  tunnel: cluster{"Ch Name":string, "Boolean":bool} {"Ch Name"="", "Boolean"=FALSE} ("Cluster") -> [w76]
                  tunnel: w56 -> [w75] mode=indexing
                  tunnel: w60 -> [w73] mode=indexing
                  tunnel: [w70] -> w63 mode=indexing
                  n485 = Unbundle By Name(w75) -> ("Ch Name"=w74:string)
                  n486 = Greater?(x=w73, y=0.5) -> (0:w71:bool)
                  n487 = Bundle By Name(cluster=w76, "Ch Name"=w74, "Boolean"=w71) -> (w70:cluster{"Ch Name":string, "Boolean":bool})
                }
                n488 = local write "Rig_Control"(w63) -> ()
              }
              frame False {
              }
            }
          }
          frame #1 {
            w91 = 300 ("y")
            n489 = global read "Trav_pos_global.vi" "Sync to server now"() -> (w77:bool)
            n490 = Quotient & Remainder(x=w93, y=86400) -> (x-y*floor(x/y)=w94:i32)  [unwired: 1 out]
            n491 = Quotient & Remainder(x=w93, y=21600) -> (x-y*floor(x/y)=w90:i32)  [unwired: 1 out]
            n492 = Equal?(x=w94, y=w91) -> (x = y?=w88:bool)
            n493 = Equal?(x=w91, y=w90) -> (x = y?=w89:bool)
            n494 = Or(x=w88, y=w89) -> (x .or. y?=w81:bool)
            n495 = Select(t=3 ("Months of History to backup"), s=w88, f=1) -> (s? t:f=w85:i32)
            n496 = global read "Preference_global.vi" "Server Comms"() -> (w83:T41)
            n497 = Equal?(x=w83, y=Server_Comms."Server Link Healthy" ("Server Comms")) -> (x = y?=w82:bool)
            n498 = And(x=w81, y=w82) -> (x .and. y?=w79:bool)
            n499 = Compound Arithmetic op=OR(w77, "Sync to server now", w79) -> (w78:bool)
            n500 = case shown="True" w78 {
              tunnel: w85 -> [_ w96]
              frame False {
              }
              frame True {
                n501 = stacked-sequence {
                  tunnel: w96 -> [w99 _]
                  frame #0 {
                    w97 = TRUE  # Check Updates on Server?
                    w98 = TRUE  # Get all Server Files
                    n502 = call "Backup_Client.vi"("Check Updates on Server?"=w97, "Get all Server Files"=w98, "Months of History to backup"=w99) -> ()  [unwired: 1 out]
                  }
                  frame #1 {
                    w100 = FALSE ("Sync to server now")
                    n503 = local write "Sync to server now"(w100) -> ()
                    n504 = global write "Trav_pos_global.vi" "Sync to server now"(w100) -> ()
                  }
                }
              }
            }
          }
          frame #2 {
            n505 = while {
              shift-right: [w108] -> _
              shift-left: "Start" -> [w110]
              tunnel: w101 -> [w107]
              shift-right: [w106] -> _
              shift-left: _ -> [w105]
              shift-right: [w104] -> _
              shift-left: _ -> [w103]
              stop <- w109 continue-if-true
              n506 = case shown="\"Run monitor\"" w110 {
                selector: w110 -> [w115 _ _ _ _ _ _ _]
                tunnel: [FALSE TRUE TRUE TRUE TRUE FALSE FALSE FALSE] -> w109
                tunnel: ["End" w123 w135 w144 w153 "End" "End" "End"] -> w108
                tunnel: w107 -> [_ _ w133 _ _ _ _ _]
                tunnel: [w112 w122 w129 w140 w158 w211 refnum<vi> refnum ("type specifier VI Refnum (for type only)") w265] -> w106
                tunnel: w105 -> [w112 w122 w129 w140 w158 w190 w246 w265]
                tunnel: [w111 w121 w128 w139 w149 w193 w243 w264] -> w104
                tunnel: w103 -> [w111 w121 w128 w139 w149 _ w243 w264]
                frame "No Match", Default {
                  n507 = Current VI's Path() -> (path=w120:path)
                  n508 = Format Into String(format string="The Case\"%s\" was not Matched\nin VI named\n'%s\"" ("Format String"), w115, w120) -> (resulting string=w117:string)  [unwired: 2 in, 1 out]
                  n509 = One Button Dialog(message=w117, button name ("OK")="STOP") -> (true=w119:bool)
                  n510 = Stop(stop? (T)=w119) -> ()
                }
                frame "Start" {
                  n511 = global read "Dynamic_call_global.ph.vi" "EnFlo Hub running?"() -> (w127:bool)
                  n512 = Select(t="Check loopcount", s=w127, f="End") -> (s? t:f=w123:string)
                }
                frame "Check loopcount" {
                  # "Only update every 10 cycles, which, based on 1000ms delay of outer loop equates to 10s sampling period"
                  # "(i MOD 10 == 0) reformulated to exclude first zero"
                  n513 = Quotient & Remainder(x=w133, y=11) -> (x-y*floor(x/y)=w131:i32)  [unwired: 1 out]
                  n514 = Equal?(x=w131, y=10) -> (x = y?=w130:bool)
                  n515 = Select(t="Check rig setup", s=w130, f="End") -> (s? t:f=w135:string)
                }
                frame "Check rig setup" {
                  n516 = global read "Preference_global.vi" "Rig Setup"() -> (w142:string)
                  n517 = Equal?(x=w142, y="EnFlo_Tunnel") -> (x = y?=w141:bool)
                  n518 = Select(t="Check LDA enabled", s=w141, f="End") -> (s? t:f=w144:string)
                }
                frame "Check LDA enabled" {
                  w155 = 0.5 ("y")
                  w151 = "LDA1:Mains_Power:Enable"
                  n519 = Build Array(w151, "LDA:System:Enable" ("Desired Ch to Read")) -> (w160:string[])
                  n520 = call "Get_Current_Scan_client.vi"("ADAM Ch Names"=w160) -> ("Numerical Values"=w159:dbl[])  [unwired: 1 in, 2 out]
                  n521 = Index Array(array=w159) -> (element #1=w156:dbl, element #2=w154:dbl)  [unwired: 2 in]
                  n522 = Greater?(x=w156, y=w155) -> (0:w152:bool)
                  n523 = Greater?(x=w154, y=w155) -> (0:w148:bool)
                  n524 = And(x=w152, y=w148) -> (x .and. y?=w150:bool)
                  n525 = case shown="False" w150 {
                    tunnel: [w166 "Run monitor"] -> w153
                    tunnel: w152 -> [w164 _]
                    tunnel: w148 -> [w165 _]
                    tunnel: w151 -> [w162 _]
                    frame False {
                      n526 = Compound Arithmetic op=AND(w165, w164) -> (w163:bool)
                      n527 = case shown="True" w164 {
                        tunnel: ["End" w170] -> w166
                        tunnel: w163 -> [_ w169]
                        tunnel: w162 -> [_ w168]
                        frame False {
                        }
                        frame True {
                          n528 = case shown="False" w169 {
                            tunnel: ["End" "Turn Off Lasers" ("t")] -> w170
                            tunnel: w168 -> [w172 _]
                            frame False {
                              n529 = Build Array(w172) -> (w174:string[])
                              n530 = Build Array(0.0 ("y")) -> (w175:dbl[])
                              n531 = call "ASYNC_Adam_client.vi"("Values"=w175, "Channel Names"=w174) -> ()  [unwired: 1 in, 2 out]
                            }
                            frame True {
                            }
                          }
                        }
                      }
                    }
                    frame True {
                    }
                  }
                }
                frame "Run monitor" {
                  w183 = errorcluster {"status"=FALSE, "code"=0, "source"=""} ("error in (no error)")
                  w193 = string[] ["LDA Laser:Green:Power (mW)", "LDA Laser:Green:LDD current (A)", "LDA Laser:Green:TEC drive (V)", "LDA Laser:Green:TEC temp. (degC)", "LDA Laser:Green:SHG heater (degC)", "LDA Laser:Green:BRF heater (degC)", "LDA Laser:Blue:Power (mW)", "LDA Laser:Blue:LDD current (A)", "LDA Laser:Blue:TEC drive (V)", "LDA Laser:Blue:TEC temp. (degC)", "LDA Laser:Blue:SHG heater (degC)", "LDA Laser:Blue:BRF heater (degC)"]
                  w208 = TRUE  # Don't Bother with check?
                  # "Call by reference to prevent loading of sub-hierarchy for rigs not using LDA. Treating the reference opening in this manner means it only ever has to be done once, and only if all checks are passed."
                  n532 = call-by-ref "Start Asynchronous Call"(reference=w190, error in=w183) -> (error out=w191:errorcluster)  [unwired: 2 in, 5 out]
                  n533 = call-by-ref "Wait On Asynchronous Call"(reference=w190, error in=w183) -> (reference out=w188:refnum<vi>, error out=w192:errorcluster, "GREEN LASER"=w187:T62, "BLUE LASER"=w186:T62, "Initialisation error"=w185:errorcluster, "IO error (first)"=w184:errorcluster)  [unwired: 2 in]
                  n534 = Merge Errors(w191, w192) -> (w189:errorcluster)
                  n535 = case shown="Error" w189 {
                    selector: w189 -> [w223 _]
                    tunnel: [w224 w230] -> w211
                    tunnel: w188 -> [w224 _]
                    tunnel: [w223 w229] -> _
                    tunnel: [w222 w225] -> w210
                    tunnel: [w221 w226] -> w209
                    tunnel: [w220 w228] -> w182
                    tunnel: [w219 w227] -> w181
                    tunnel: w187 -> [w222 _]
                    tunnel: w186 -> [w221 _]
                    tunnel: w185 -> [w220 _]
                    tunnel: w184 -> [w219 _]
                    frame No Error {
                    }
                    frame Error {
                      n536 = Current VI's Path() -> (path=w239:path)
                      n537 = Strip Path(path=w239) -> (stripped path=w240:path)  [unwired: 1 out]
                      n538 = Build Path(base path=w240, name or relative path=path "Anemometry Sub Vis/LDA/Coherent/Lasers monitor ONESHOT.vi") -> (appended path=w237:path)
                      n539 = Open VI Reference(type specifier VI Refnum (for type only)=refnum<vi> refnum, vi path=w237, options=256, error in (no error)=errorcluster {"status"=FALSE, "code"=0, "source"=""}) -> (vi reference=w232:refnum<vi>, error out=w233:errorcluster)  [unwired: 2 in]
                      n540 = call-by-ref "Start Asynchronous Call"(reference=w232, error in=w233) -> (error out=w234:errorcluster)  [unwired: 2 in, 5 out]
                      n541 = call-by-ref "Wait On Asynchronous Call"(reference=w232, error in=w233) -> (reference out=w230:refnum<vi>, error out=w231:errorcluster, "GREEN LASER"=w225:T62, "BLUE LASER"=w226:T62, "Initialisation error"=w228:errorcluster, "IO error (first)"=w227:errorcluster)  [unwired: 2 in]
                      n542 = Merge Errors(w234, w231) -> (w229:errorcluster)
                    }
                  }
                  n543 = Unbundle By Name(w210) -> ("Power (mW)"=w207:sgl, "LDD current (A)"=w206:sgl, "TEC drive (V)"=w205:sgl, "TEC temp. (degC)"=w204:sgl, "SHG heater (degC)"=w203:sgl, "BRF heater (degC)"=w202:sgl)
                  n544 = Unbundle By Name(w209) -> ("Power (mW)"=w201:sgl, "LDD current (A)"=w200:sgl, "TEC drive (V)"=w199:sgl, "TEC temp. (degC)"=w198:sgl, "SHG heater (degC)"=w197:sgl, "BRF heater (degC)"=w196:sgl)
                  n545 = Build Array(w207, w206, w205, w204, w203, w202, w201, w200, w199, w198, w197, w196) -> (w195:sgl[])
                  n546 = Merge Errors(w182, w181) -> (w180:errorcluster)
                  n547 = for {
                    tunnel: w193 -> [w217] mode=indexing
                    tunnel: w195 -> [w216] mode=indexing
                    tunnel: [w214] -> w194 mode=indexing
                    n548 = To Double Precision Float(number=w216) -> (double precision float=w215:dbl)
                    n549 = Bundle By Name(cluster=T42 {"Channel Name"="", "New Value"=0.0} ("Update Scan Value Cluster"), "Channel Name"=w217, "New Value"=w215) -> (w214:T42)
                  }
                  n550 = call "EnFlo_Error_Handler.vi"("error in (no error)"=w180, "Error Type"="LDA1_Monitor", "Dialog Box (T)"=FALSE) -> ()  [unwired: 3 out]
                  n551 = call "Update_Current_Value_client.vi"("Don't Bother with check?"=w208, "Update array in"=w194) -> ()
                }
                frame "Turn Off Lasers" {
                  w245 = TRUE  # Don't Bother with check?
                  w249 = FALSE ("Green Laser on")
                  n552 = for {
                    tunnel: w243 -> [w262] mode=indexing
                    tunnel: [w261] -> w244 mode=indexing
                    n553 = Bundle By Name(cluster=T42 {"Channel Name"="", "New Value"=0.0} ("Update Scan Value Cluster"), "Channel Name"=w262, "New Value"=nan) -> (w261:T42)
                  }
                  n554 = Current VI's Path() -> (path=w253:path)
                  n555 = Strip Path(path=w253) -> (stripped path=w254:path)  [unwired: 1 out]
                  n556 = call "Update_Current_Value_client.vi"("Don't Bother with check?"=w245, "Update array in"=w244) -> ()
                  n557 = Close Reference(reference=w246) -> ()  [unwired: 1 in, 1 out]
                  n558 = Build Path(base path=w254, name or relative path=path "Anemometry Sub Vis/LDA/Coherent/Laser power on,off (simple).vi") -> (appended path=w251:path)
                  n559 = Open VI Reference(type specifier VI Refnum (for type only)=refnum<vi> refnum, vi path=w251, error in (no error)=errorcluster {"status"=FALSE, "code"=0, "source"=""}) -> (vi reference=w257:refnum<vi>, error out=w256:errorcluster)  [unwired: 3 in]
                  n560 = call-by-ref "?"(reference=w257, error in=w256, "Green Laser on"=w249, "Blue Laser on"=w249) -> (reference out=w248:refnum<vi>, error out=w247:errorcluster)  [unwired: 3 out]
                  n561 = Close Reference(reference=w248, error in (no error)=w247) -> ()  [unwired: 1 out]
                }
                frame "End" {
                }
              }
            }
          }
        }
        n562 = Wait (ms)(milliseconds to wait=u32 1000) -> ()  [unwired: 1 out]
      }
    }
  }
  n563 = call "Last_modified_date.vi"("Update Now"=TRUE) -> ("RevisionString"=w2:string)  [unwired: 1 out]
  n564 = global write "Meas_global.vi" "ProgRevisionInfo"(w2) -> ()
